vi "运维调试_CODMn.vi"() -> ()   [LabVIEW 2016, in "斯坦道CODMn新电路板.lvlib"]
uses:
  <vilib>/Utility/miscctls.llb/LVPointTypeDef.ctl
  <vilib>/Waveform/WDTFileIO.llb/Read Waveform from File.vi
  <vilib>/Utility/config.llb/NI_LVConfig.lvlib
  <vilib>/ptbypt/NI_PtbyPt.lvlib
panel:
  out "权限等级":string
  out "总步数":i32
  out "滑动杆":u8(slide) caption="测试进度" scale=0.0..100.0
  in  "参数查询":bool
  in  "仪器校准":bool
  out "仪器版本号":string
  in  "试剂余量设置":bool
  out "试剂余量显示":sgl[][](graph)
  in  "公式切换阈值滴定数(0~9999)":dbl
  out "X0":u16
  in  "平台反控标样校准":enum16{"标液1", "标液2", "标液3"}(ring)
  in  "平台反控校准量程":enum16{"低量程1", "低量程2", "高量程1", "高量程2"}(ring)
  out "注射泵保温温度":sgl format="%#.2g"
  out "量程参数显示":T1 {"(高->低)" format="%#.6g"; "阈值(低->高)" format="%#.6g"; "下限" format="%#.6g"; "上限" format="%#.6g"}
  in  "历史波形 2":bool
  in  "返回 3":bool
  out "时间-温度":u16[](array[numeric]) caption="数组"
  out "温度波形时间":timestamp
  out "ORP滴定曲线 2":u16[](graph)
  in  "历史波形":bool
  in  "返回 2":bool
  out "滴定数-ORP值":u16[](array[numeric]) caption="数组"
  out "波形时间":timestamp
  out "ORP滴定曲线":u16[](graph)
  in  "滴定曲线":bool
  out "终点滴定数":sgl format="%#.2f"
  in  "量程参数设置":bool
  out "单位:":T2(ring)
  out "运行状态":T3 {"数据时间:" format="%<%y/%m/%d %H:%M:%S>T"; "仪器时间:" format="%<%y/%m/%d %H:%M:%S>T"}
  out "模块版本号":string
  in  "模型选择":cluster{"参数":u8, "测量模式":u8, "量程":u8}
  in  "校准完毕":bool
  in  "校准按钮":T4
  in  "曲线模型":T5={"标液浓度1"=0.0, "测量吸光度1"=0.0, "样品1启用"=FALSE, "标液浓度2"=0.0, "测量吸光度2"=0.0, "样品2启用"=FALSE, "标液浓度3"=0.0, "测量吸光度3"=0.0, "样品3启用"=FALSE, "标液浓度4"=0.0, "测量吸光度4"=0.0, "样品4启用"=FALSE, "标液浓度5"=0.0, "测量吸光度5"=0.0, "样品5启用"=FALSE, "模型"=enum."线性", "method"=enum."最小二乘", "精度"=7.0, "XY图"=[], "拟合公式"="", "r^2"=0.0, "零点校准时间"=timestamp(0 s since 1904-01-01), "标液校准时间1"=timestamp(0 s since 1904-01-01), "标液校准时间2"=timestamp(0 s since 1904-01-01), "标液校准时间3"=timestamp(0 s since 1904-01-01), "标液校准时间4"=timestamp(0 s since 1904-01-01)} {"标液校准时间4" format="%<%Y/%m/%d %H:%M:%S>T"; "标液校准时间3" format="%<%Y/%m/%d %H:%M:%S>T"; "标液校准时间2" format="%<%Y/%m/%d %H:%M:%S>T"; "标液校准时间1" format="%<%Y/%m/%d %H:%M:%S>T"; "零点校准时间" format="%<%Y/%m/%d %H:%M:%S>T"; "r^2" format="%.7g"; "标液浓度5" format="%#.2f"; "测量吸光度5" format="%#.0f"; "标液浓度4" format="%#.2f"; "测量吸光度4" format="%#.0f"; "标液浓度3" format="%#.2f"; "测量吸光度3" format="%#.0f"; "标液浓度2" format="%#.2f"; "测量吸光度2" format="%#.0f"; "测量吸光度1" format="%#.0f"; "标液浓度1" format="%#.2f"}
  out "公式、校准输出":T6={"公式"={"X^2"=0.0, "X"=nan, "B"=nan}, "校准"={"校准？"=FALSE, "校准点1-5"=0, "校准浓度"=0.0}}
  out "当前步骤剩余时间":sgl format="%#.2f"
  out "加热实时温度":sgl format="%#.2f"
  out "ORP值":sgl format="%#.2f"
  in  "布尔":bool
  in  "关键参数设置":bool
  in  "流程固件":bool
  in  "模块启用":bool
  in  "串口设置":bool
  in  "公式单个写入":bool
  in  "流程路径":path=path "C:/Users/STD/Documents/斯坦道流程文件/流程.xml"
  out "字符串":string
  out "运行时间":sgl format="%#.2g"
  out "环境湿度":sgl format="%#.2g"
  out "环境温度":sgl format="%#.2g"
  out "固件版本号":string
  in  "数组":string[](array[string])
  in  "量程切换阈值写入":bool
  in  "量程切换阈值读取":bool
  in  "参数下拉列表":enum16{"CODMn"}(ring)
  in  "量程下拉列表":enum16{"低量程1", "低量程2", "高量程1", "高量程2"}(ring)
  in  "测量模式下拉列表":T7(ring)=enum."水样测量"
  in  "公式":cluster{"X^2":dbl, "X":dbl, "b":dbl}
  in  "写公式":bool
  in  "读公式":bool
  in  "返回":bool
  in  "设置":bool
  out "集成报警信息":string
  in  "定时启动":cluster{"启动":bool, "控制命令":T8, "测量参数":T9}(xcontrol)
  in  "停止":bool
  in  "手动启动":bool
  in  "单步测试":bool
  out "当前滴定数":sgl format="%#.2f"
  out "K":sgl format="%#.2f"
  out "B":sgl format="%#.2f"
  out "A":sgl format="%#.2f"
  out "多列列表框":i32(listbox)
  # "."
  # "校准时间"
  # "标液浓度"
  # "滴定数显示"
  # "标液1"
  # "标液2"
  # "标液3"
  # "零点"
  # "跨度"
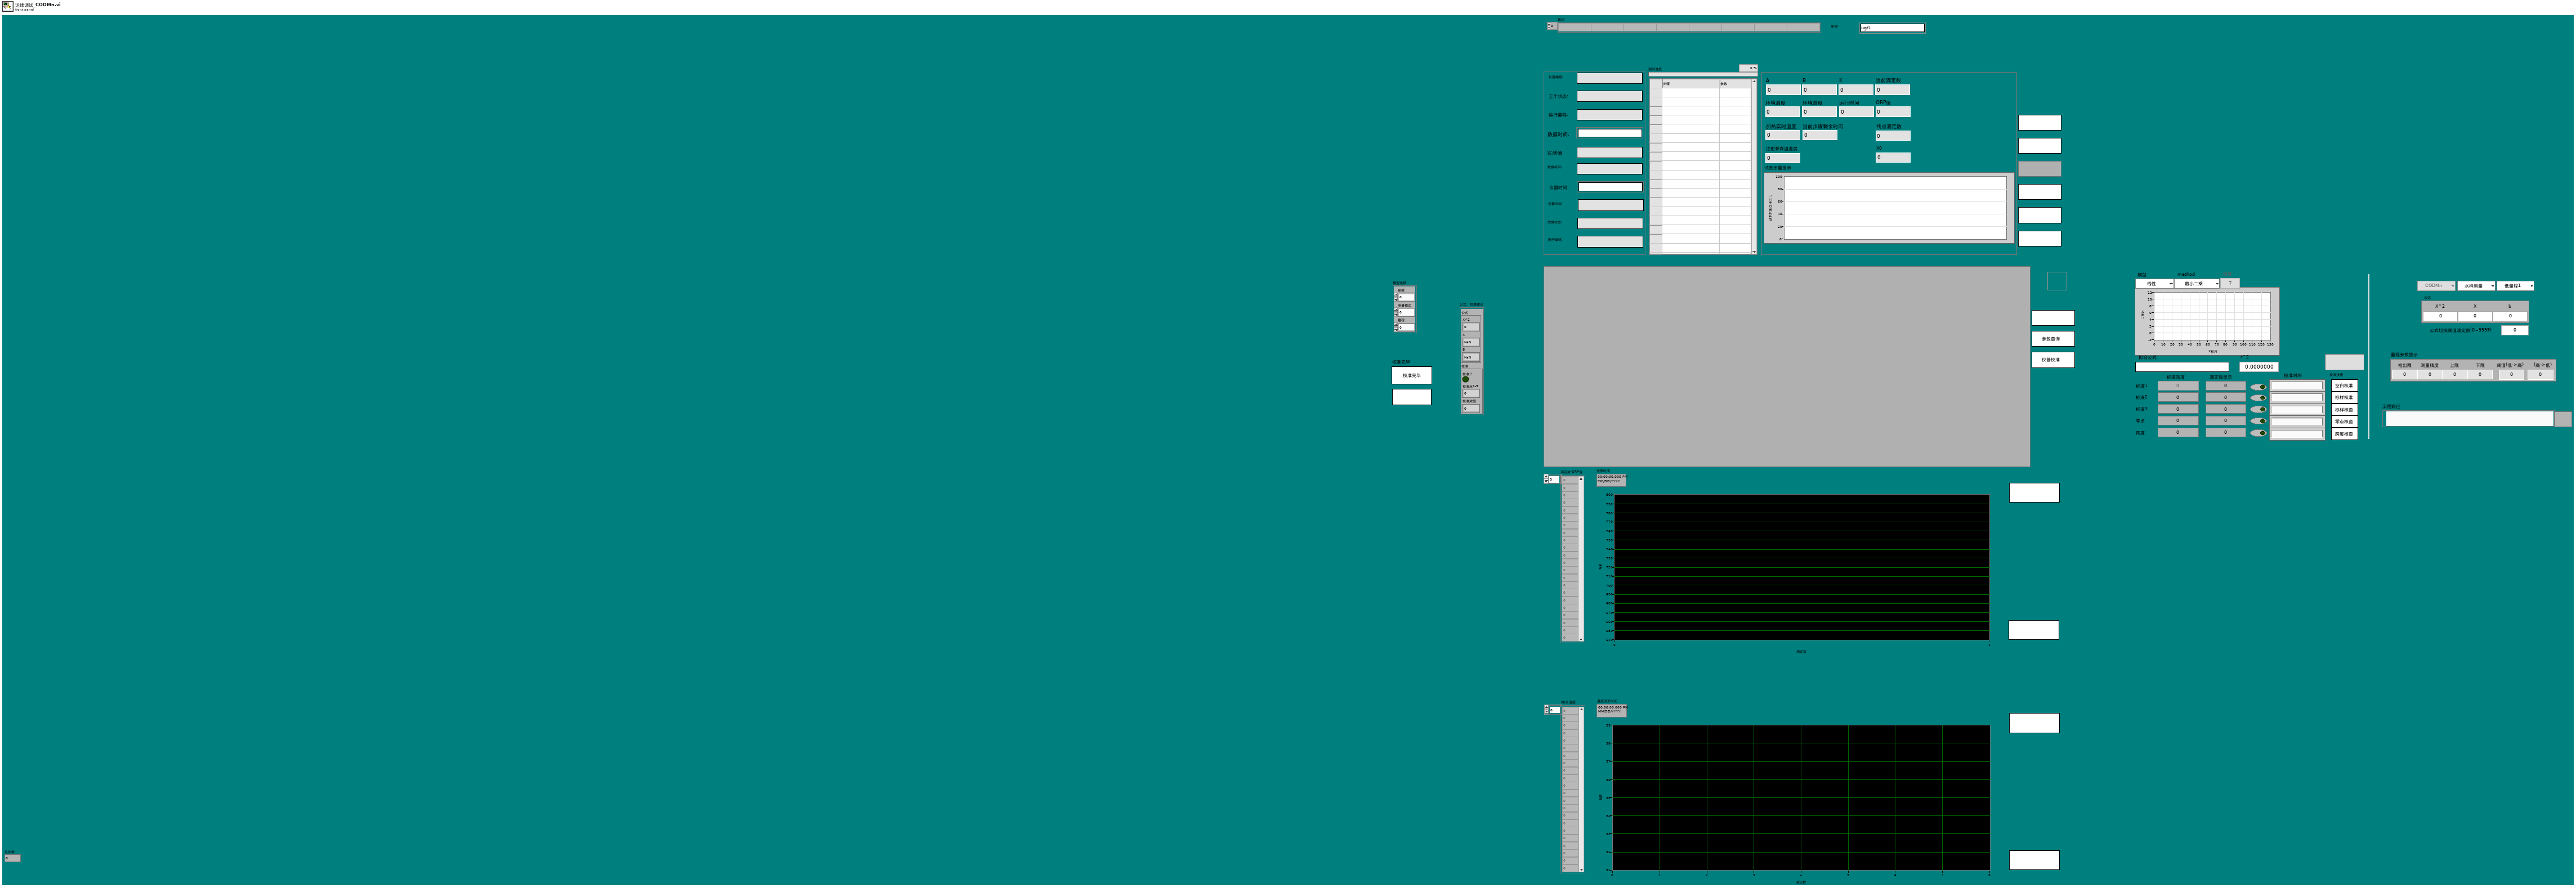
[diagram p1: front panel]
types:
  T1 = cluster{"检出限":dbl, "测量精度":dbl, "上限":dbl, "下限":dbl, "阈值(低->高)":dbl, "(高->低)":dbl}
  T2 = enum16{"ug/L", "mg/L", "ppm", "mg/m3", "cm", "ppb", "ug/m3", "%", "nmol/mol", "umol/mol", "MPN/L", "MPN/100ml", "ng/m3", "NTU", "无量纲", "ms/cm", "us/cm", "℃", "mV", "万个/L"}
  T3 = cluster{"仪器编号:":string, "工作状态:":string, "运行量程: ":string, "数据时间:":timestamp, "实测值:":string, "数据标识: ":string, "仪器时间:":timestamp, "告警状态: ":string, "故障状态:  ":string, "因子编码:":string}
  T4 = cluster{"校准1":bool, "校准2":bool, "校准3":bool, "校准4":bool, "校准5":bool}
  T5 = cluster{"标液浓度1":dbl, "测量吸光度1":dbl, "样品1启用":bool, "标液浓度2":dbl, "测量吸光度2":dbl, "样品2启用":bool, "标液浓度3":dbl, "测量吸光度3":dbl, "样品3启用":bool, "标液浓度4":dbl, "测量吸光度4":dbl, "样品4启用":bool, "标液浓度5":dbl, "测量吸光度5":dbl, "样品5启用":bool, "模型":enum32{"线性", "多项式"}, "method":enum16{"最小二乘", "最小绝对残差", "Bisquare"}, "精度":dbl, "XY图":cluster{"X Values":dbl[], "Y Values":dbl[]}[], "拟合公式":string, "r^2":dbl, "零点校准时间":timestamp, "标液校准时间1":timestamp, "标液校准时间2":timestamp, "标液校准时间3":timestamp, "标液校准时间4":timestamp}
  T6 = cluster{"公式":cluster{"X^2":dbl, "X":dbl, "B":dbl}, "校准":cluster{"校准？":bool, "校准点1-5":u16, "校准浓度":dbl}}
  T7 = enum16{"", "水样测量", "标样核查", "零点核查", "跨度核查", "空白测试", "平行样测试", "加标回收"}
  T8 = typedef "定时设置.xctl/国标控制命令.ctl" = enum16{"启动测量", "标样核查", "零点核查", "跨度核查", "空白测试", "平行样测试", "加标回收", "空白校准", "标样校准", "初始化（清洗）", "停止测试", "仪器重启", "校时", "模式设置", "测量间隔设置"}
  T9 = typedef "定时设置.xctl/测量参数.ctl" = u16
  T10 = cluster{"曲线模型":cluster{"标液浓度1":dbl, "测量吸光度1":dbl, "样品1启用":bool, "标液浓度2":dbl, "测量吸光度2":dbl, "样品2启用":bool, "标液浓度3":dbl, "测量吸光度3":dbl, "样品3启用":bool, "标液浓度4":dbl, "测量吸光度4":dbl, "样品4启用":bool, "标液浓度5":dbl, "测量吸光度5":dbl, "样品5启用":bool, "模型":enum32{"线性", "多项式"}, "method":enum16{"最小二乘", "最小绝对残差", "Bisquare"}, "精度":dbl, "XY图":cluster{"X Values":dbl[], "Y Values":dbl[]}[], "拟合公式":string, "r^2":dbl, "零点校准时间":timestamp, "标液校准时间1":timestamp, "标液校准时间2":timestamp, "标液校准时间3":timestamp, "标液校准时间4":timestamp}, "Polynomial Coefficients":dbl[]}
  T11 = cluster{"Major":u16, "Minor":u16, "Fix":u16, "Build":u16}
  T12 = typedef "NI_LVConfig.lvlib/Config Data RefNum.ctl" = refnum<k1>
  T13 = typedef "LVPointTypeDef.ctl" = cluster{"Horizontal":i16, "Vertical":i16}
  T14 = enum32{"Bad", "Idle", "Run top level", "Running"}
  T15 = cluster{"Polynomial Coefficients[0]":dbl, "Polynomial Coefficients[1]":dbl, "Polynomial Coefficients[2]":dbl}
  T16 = cluster{"检出限":dbl, "测量精度":dbl, "上限":dbl, "下限":dbl, "阈值（低->高）":dbl, "阈值（高->低）":dbl}
  T17 = cluster{"系统时间":timestamp, "工作状态":u16, "测量模式":enum16{"待机", "连续模式", "周期模式", "定点模式", "受控模式", "手动模式"}, "告警代码":u16, "故障代码":u16, "日志代码":u16, "软件版本":u16, "A":sgl, "B":sgl, "K":sgl, "当前滴定数":sgl, "T":sgl, "H":sgl, "id":u16, "flowid":u16, "量程":u16, "加热实时温度":sgl, "当前ORP值":sgl, "运行时间":sgl, "当前步骤剩余时间":sgl, "结束滴定数":sgl, "注射泵保温温度":sgl, "匹配滴定数X0":u16, "X^2":sgl, "X":sgl, "B 2":sgl}
  T18 = cluster{"因子编码":u32, "单位":u16, "标样参考值":sgl, "水样数据时间":timestamp, "水样实测值":sgl, "水样数据标识":string, "标样数据时间":timestamp, "标样实测值":sgl, "标样数据标识":string, "空白数据时间":timestamp, "空白实测值":sgl, "空白数据标识":string, "零点核查数据时间":timestamp, "零点核查实测值":sgl, "零点核查数据标识":string, "跨度核查数据时间":timestamp, "跨度核查实测值":sgl, "跨度核查数据标识":string, "加标回收数据时间":timestamp, "加标回收实测值":sgl, "加标回收数据标识":string, "平行样数据时间":timestamp, "平行样实测值":sgl, "平行样数据标识":string, "F0":sgl, "F1":sgl, "F2":sgl, "F3":sgl, "F4":sgl, "F5":sgl, "F6":sgl, "F7":sgl, "温度":sgl, "湿度":sgl, "X值":sgl, "fidrange":u16}
  T19 = cluster{"时间标识":timestamp, "设备":string, "日志信息":string, "流程参数":string}
  T20 = cluster{"时间标识":timestamp, "设备":string, "日志信息":string, "备注":string}
  T21 = typedef "LVRowAndColumnUnsignedTypeDef.ctl" = cluster{"Row":u32, "Column":u32}
  T22 = enum8{"Enabled", "Disabled", "Disabled and Grayed Out"}
  T23 = cluster{"时间源选择":enum16{"系统时间源", "仪器时间源"}, "外部时间源":timestamp}
  T24 = enum16{"空闲", "水样测试", "标样核查", "零点核查", "跨度核查", "空白测试", "平行样测试", "加标回收", "空白校准", "标样校准", "初始化（清洗）"}
  T25 = cluster{"站号":u16, "量程切换":enum32{"H", "L", "AUTO"}, "控制命令":u16, "模式设置":enum16{"待机", "连续模式", "周期模式", "定点模式", "受控模式", "手动模式"}, "测量间隔":u16}
  T26 = cluster{"参数下拉列表":enum16{"CODMn"}, "测量模式下拉列表":enum16{"", "水样测量", "标样核查", "零点核查", "跨度核查", "空白测试", "平行样测试", "加标回收"}, "量程下拉列表":enum16{"低量程1", "低量程2", "高量程1", "高量程2"}}
  T27 = cluster{"测量量程":dbl, "测量精度":dbl, "测量间隔":dbl, "消解温度":dbl, "消解时长":dbl, "空白校准时间":timestamp, "曲线截距":dbl, "曲线斜率":dbl, "测量检出限":dbl, "测量信号值":dbl, "线性相关系数":dbl, "二次多项式系数":dbl, "标样校准时间":timestamp, "稀释倍数":dbl, "三项式系数":dbl, "空白标定系数":dbl, "量程系数":dbl, "F0/ORPA":dbl, "F1/ORPB":dbl, "F2/ORPK":dbl, "F3":dbl, "F4":dbl, "F5":dbl, "F6":dbl, "F7":dbl, "X0/滴定数":dbl, "量程":dbl}
  T28 = typedef "量程选择控件.ctl" = enum32{"L", "H", "AUTO"}
  T29 = cluster{"水样测试量程模式":T28, "标样核查量程模式":T28, "零点核查量程模式":T28, "跨度核查量程模式":T28, "空白测试量程模式":T28, "平行样测试量程模式":T28, "加标回收量程模式":T28, "空白校准量程模式":T28, "标样校准量程模式":T28}
  T30 = cluster{"跨度值":dbl, "零点标准液浓度":dbl, "跨度标准液浓度":dbl, "标准液标准浓度":dbl}
  T31 = cluster{"水样测试量程模式":T28, "标样核查量程模式":T28, "零点核查量程模式":T28, "跨度核查量程模式":T28, "空白测试量程模式":T28, "平行样测试量程模式":T28, "加标回收量程模式":T28, "标样校准量程模式":T28, "空白校准量程模式":T28}
  T32 = cluster{"确定":bool, "跨度值":dbl, "零点标准液浓度":dbl, "跨度标准液浓度":dbl, "标准液标准浓度":dbl}
  T33 = cluster{"确定":bool, "测量量程":dbl, "测量精度":dbl, "测量间隔":dbl, "消解温度":dbl, "消解时长":dbl, "空白校准时间":timestamp, "曲线截距":dbl, "曲线斜率":dbl, "测量检出限":dbl, "测量信号值":dbl, "线性相关系数":dbl, "二次多项式系数":dbl, "标样校准时间":timestamp, "稀释倍数":dbl, "三项式系数":dbl, "空白标定系数":dbl, "量程系数":dbl, "F0/ORPA":dbl, "F1/ORPB":dbl, "F2/ORPK":dbl, "F3":dbl, "F4":dbl, "F5":dbl, "F6":dbl, "F7":dbl, "X0/滴定数":dbl, "量程":dbl}
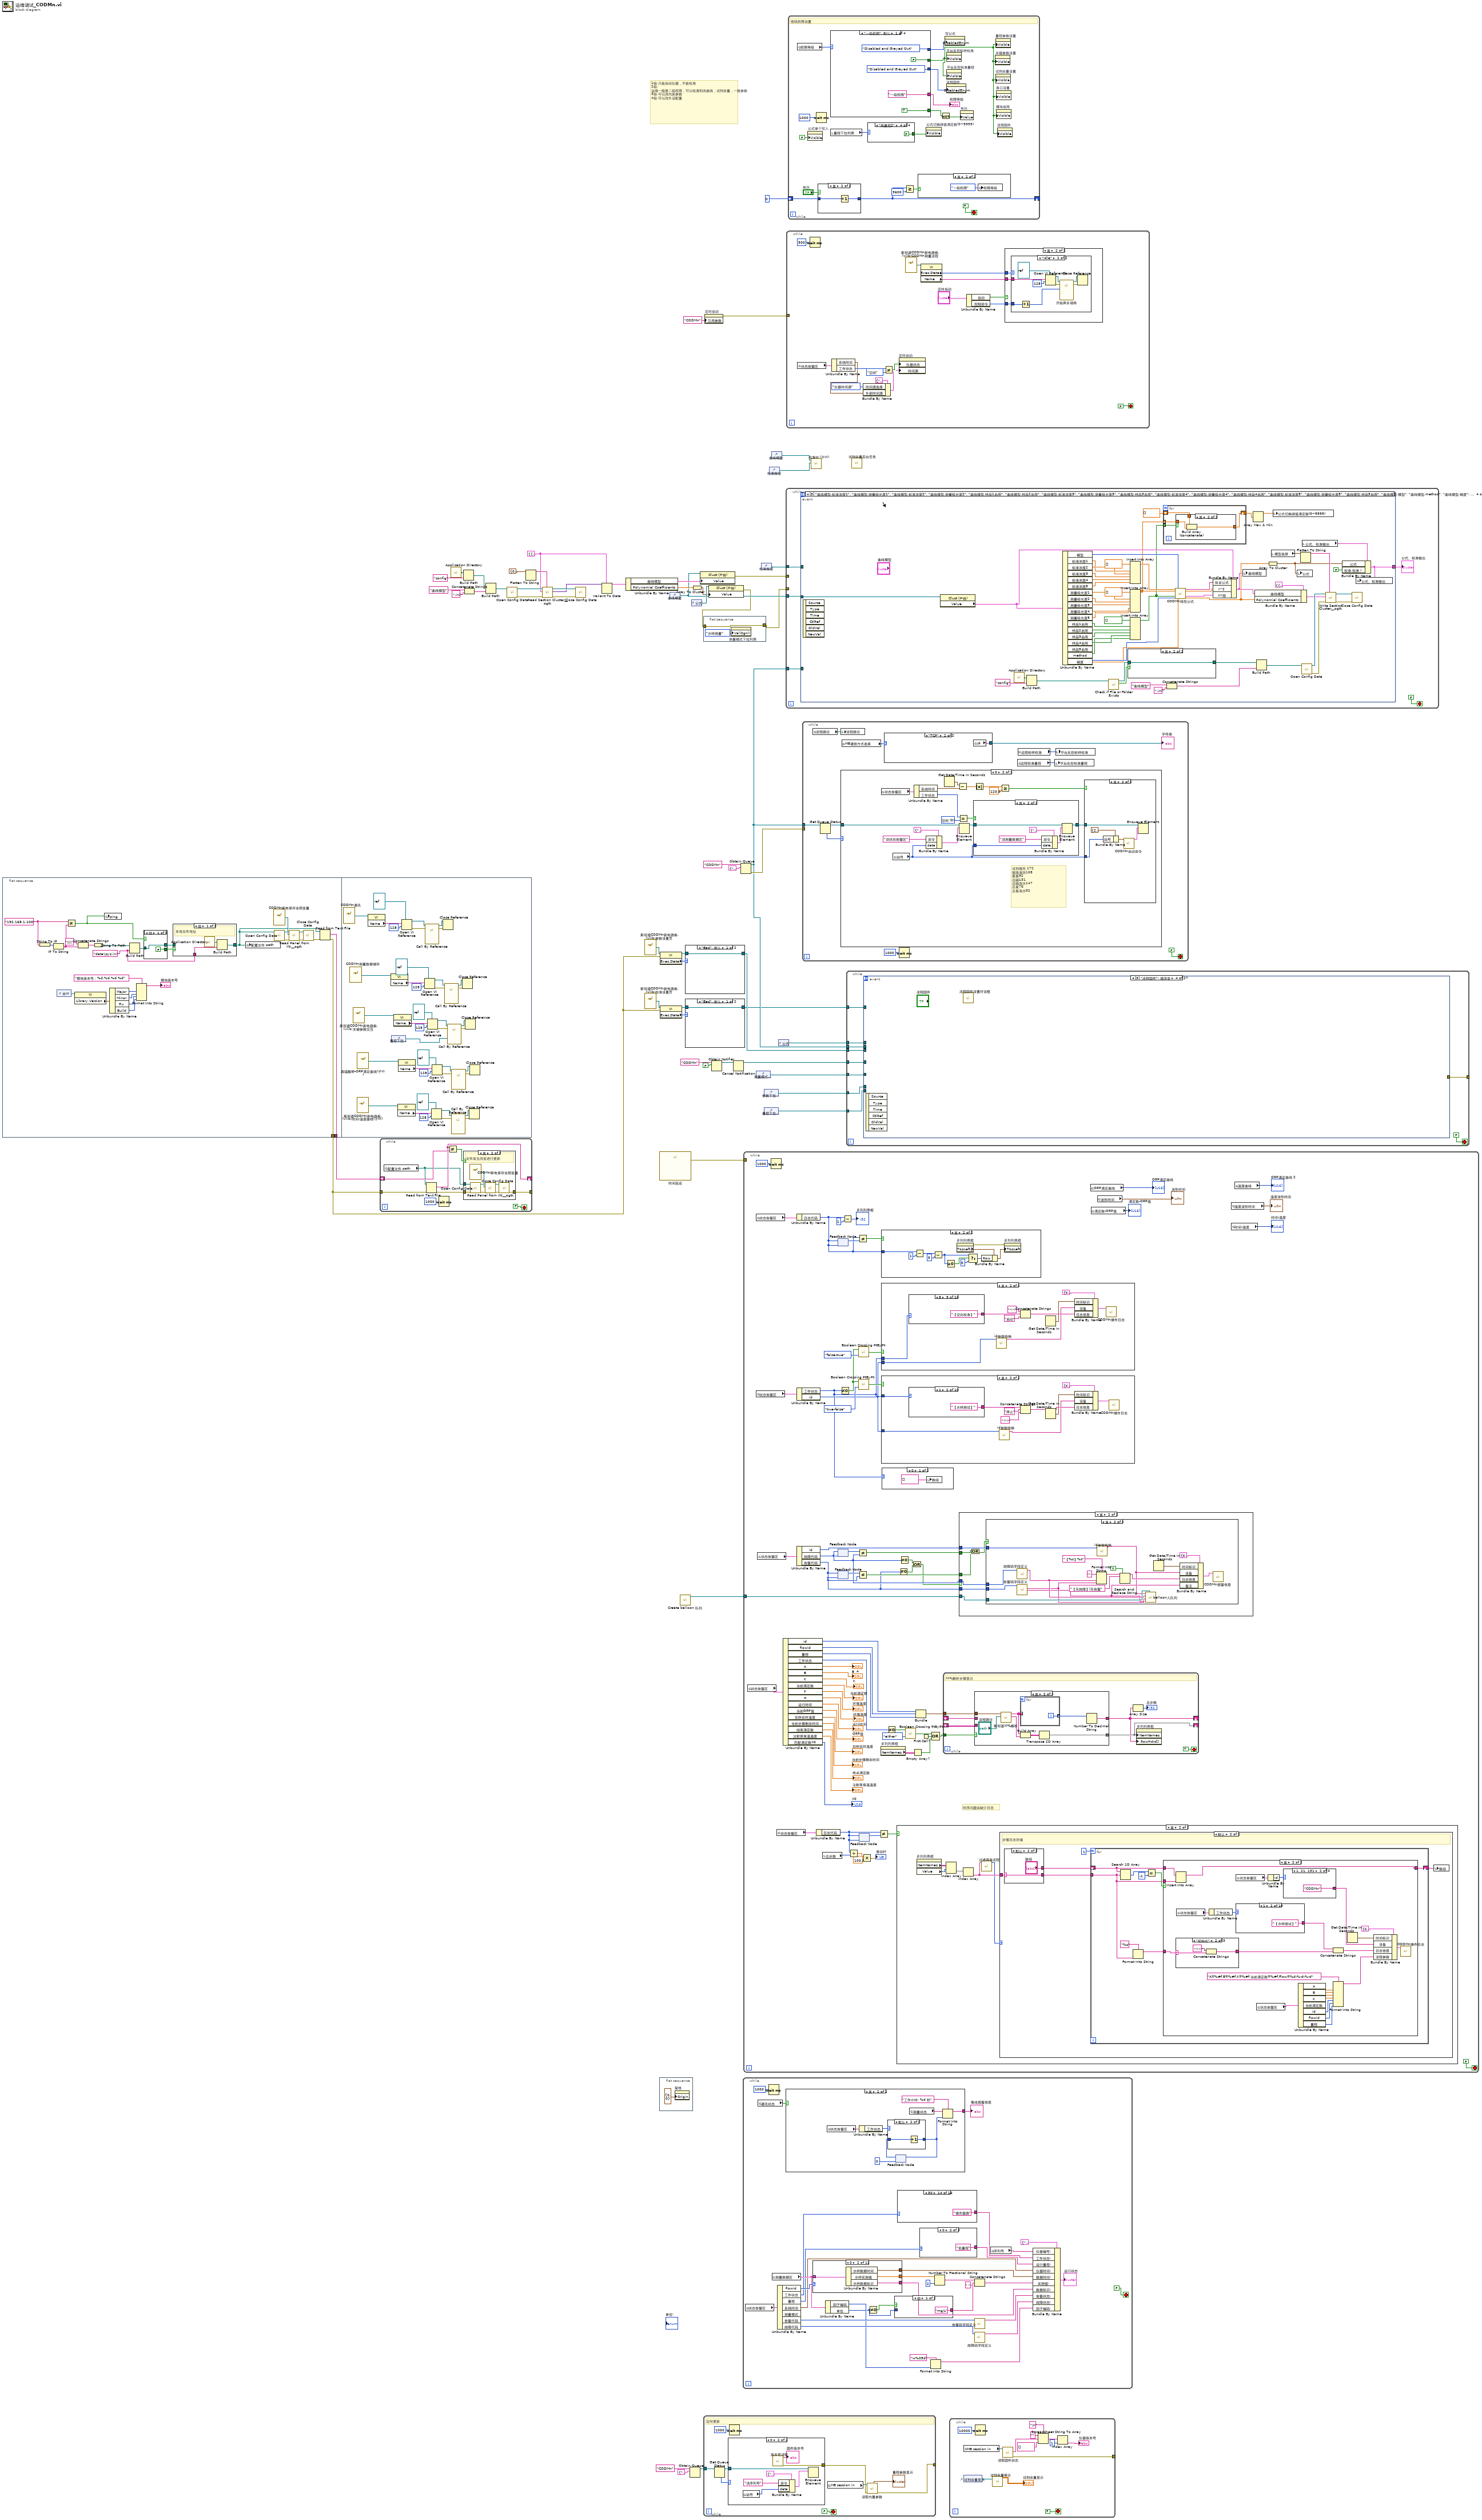
[diagram p0: block diagram]
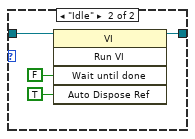
[diagram p2: hidden frame]
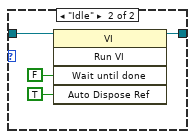
[diagram p3: hidden frame]
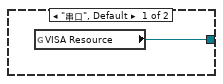
[diagram p8: hidden frame]
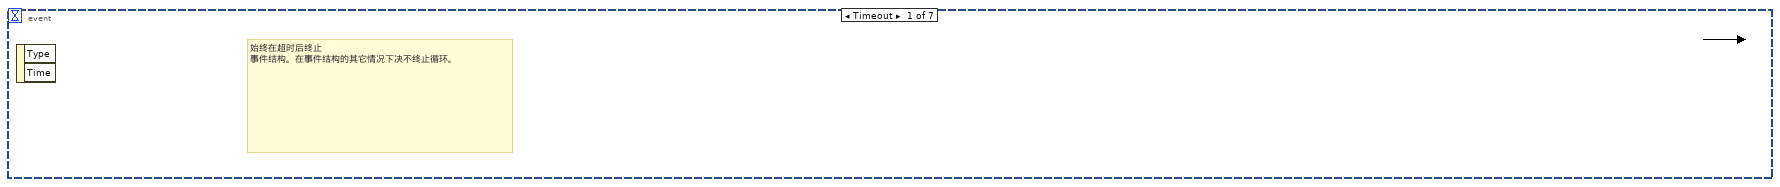
[diagram p12: hidden frame]
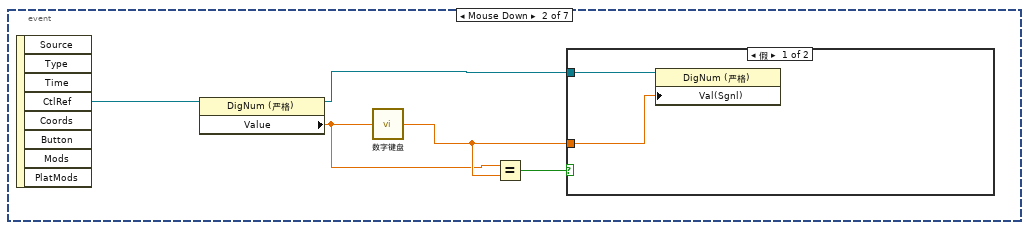
[diagram p13: hidden frame]
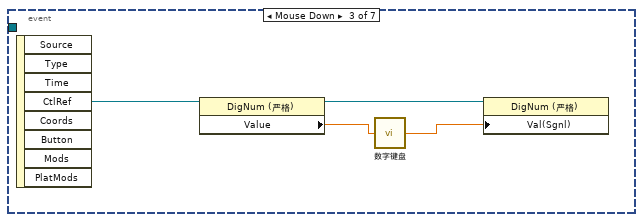
[diagram p15: hidden frame]
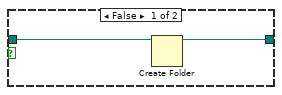
[diagram p17: hidden frame]
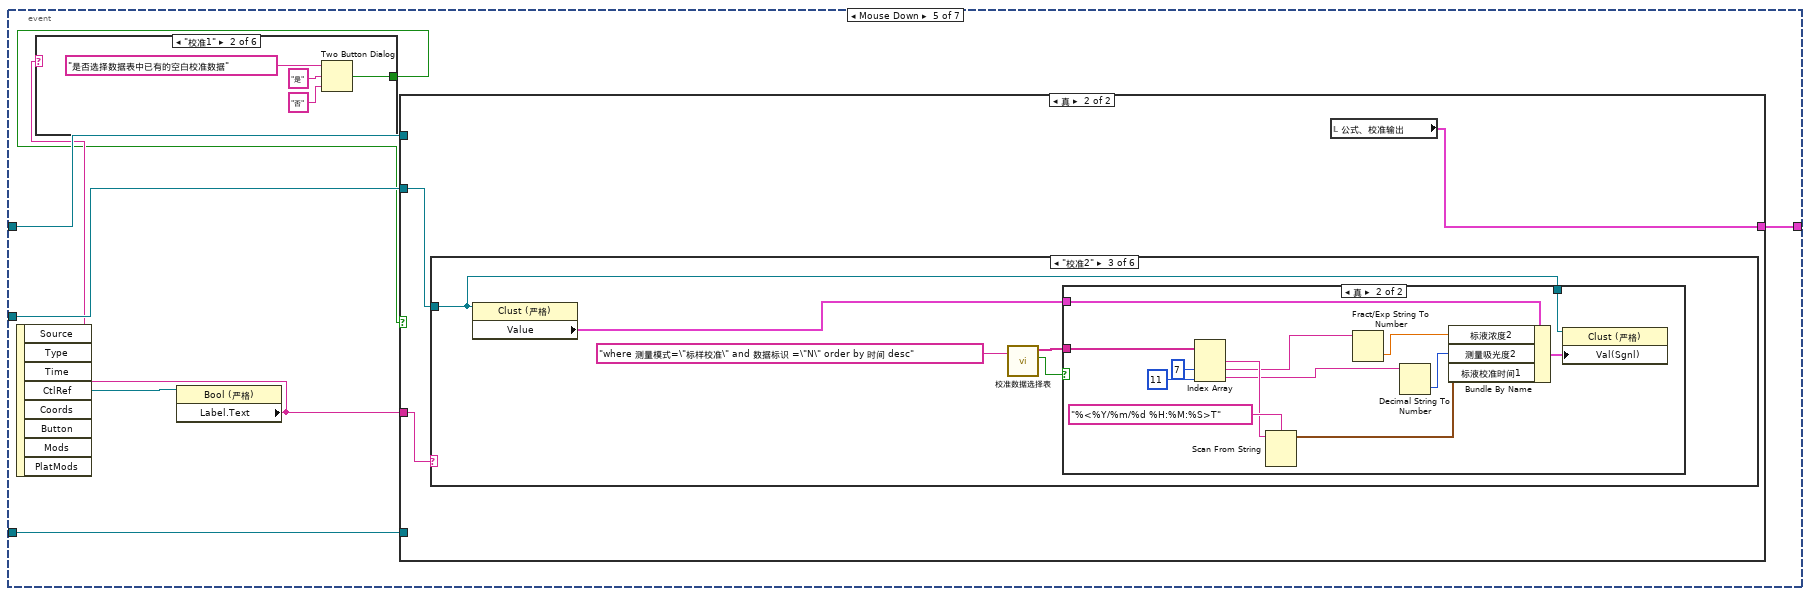
[diagram p18: hidden frame]
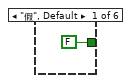
[diagram p19: hidden frame]
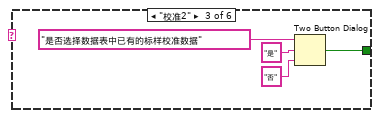
[diagram p20: hidden frame]
diagram:
  w24 = T10 {"曲线模型"={"标液浓度1"=0.0, "测量吸光度1"=0.0, "样品1启用"=FALSE, "标液浓度2"=0.0, "测量吸光度2"=0.0, "样品2启用"=FALSE, "标液浓度3"=0.0, "测量吸光度3"=0.0, "样品3启用"=FALSE, "标液浓度4"=0.0, "测量吸光度4"=0.0, "样品4启用"=FALSE, "标液浓度5"=0.0, "测量吸光度5"=0.0, "样品5启用"=FALSE, "模型"=enum."线性", "method"=enum."最小二乘", "精度"=7.0, "XY图"=[], "拟合公式"="", "r^2"=0.0, "零点校准时间"=timestamp(0 s since 1904-01-01), "标液校准时间1"=timestamp(0 s since 1904-01-01), "标液校准时间2"=timestamp(0 s since 1904-01-01), "标液校准时间3"=timestamp(0 s since 1904-01-01), "标液校准时间4"=timestamp(0 s since 1904-01-01)}, "Polynomial Coefficients"=[]} ("输出簇")
  # "1级.只能启动仪器，不能校准\n2级.运维一般是二级权限，可以校准和改曲线，试剂余量，一般参数\n3级.可以改内部参数\n4级.可以改外设配置"
  n1 = flat-sequence {
    tunnel: [w59] -> w1
    tunnel: [w58] -> w41
    frame #0 {
      w79 = "data\\sys.ini" ("名称或相对路径")
      w71 = "192.168.1.100" ("名称")
      n2 = String To IP(1:w71) -> (0:w78:u32)
      n3 = IP To String(2:w78) -> (0:w75:string)  [unwired: 1 in]
      n4 = control-ref of="本VI"() -> (w69:refnum<vi>)
      n5 = Not Equal?(x=w71, y=w75) -> (x != y?=w80:bool)
      n6 = property class="VI"(reference=w69) -> ("Library.Version"=w68:T11)  [unwired: 1 in, 2 out]
      n7 = Concatenate Strings("\\\\" ("字符串"), w75) -> (w76:string)
      n8 = String To Path(string=w76) -> (path=w70:path)
      n9 = global write "VARCODMn全局变量.vi" "ping"(w80) -> ()
      n10 = Unbundle By Name(w68) -> ("Major"=w66:u16, "Minor"=w65:u16, "Fix"=w64:u16, "Build"=w63:u16)
      n11 = Build Path(base path=w70, name or relative path=w79) -> (appended path=w74:path)
      n12 = Format Into String(format string="模块版本号：%d.%d.%d.%d" ("格式字符串"), w66, w65, w64, w63) -> (resulting string=→"模块版本号":string)  [unwired: 2 in, 1 out]
      n13 = case shown="假" w80 {
        tunnel: w74 -> [w86 w90]
        tunnel: [w86 w89] -> w73
        tunnel: [FALSE w88] -> w72
        frame False {
        }
        frame True {
          n14 = call <vilib>:"Check if File or Folder Exists.vi"("path"=w90) -> ("file or folder exists?"=w88:bool, "dup path"=w89:path)  [unwired: 8 in, 1 out]
        }
      }
      n15 = case shown="假" w72 {
        tunnel: w73 -> [_ w94]
        tunnel: [w92 w94] -> w61
        tunnel: w79 -> [w91 _]
        frame False {
          # "本地文件地址"
          n16 = call <vilib>:"Application Directory.vi"() -> ("Application Directory"=w93:path)
          n17 = Build Path(base path=w93, name or relative path=w91) -> (appended path=w92:path)
        }
        frame True {
          # "网络共享地址"
        }
      }
      n18 = global write "VARCODMn全局变量.vi" "配置文件 path"(w61) -> ()
      n19 = vi-ref "CODMn断电保存全局变量.vi"() -> (w84:refnum<vi>)
      n20 = call <vilib>:"Open Config Data.vi"("configuration file path"=w61) -> ("error out"=w82:errorcluster, "refnum"=w85:T12)  [unwired: 8 in, 1 out]
      n21 = call <userlib>:"Read Panel from INI__ogtk.vi"("error in (no error)"=w82, "VI ref"=w84, "refnum"=w85) -> ("error out"=w81:errorcluster, "refnum out"=w83:T12)  [unwired: 7 in]
      n22 = call <vilib>:"Close Config Data.vi"("error in (no error)"=w81, "refnum"=w83) -> ("error out"=w60:errorcluster)  [unwired: 8 in, 1 out]
      n23 = Read from Text File(file (use dialog)=w61, error in=w60) -> (text=w58:string, error out=w59:errorcluster)  [unwired: 2 in, 2 out]
    }
    frame #1 {
      n24 = vi-ref "CODMn通讯.vi"() -> (w103:refnum<vi>)
      n25 = vi-ref "CODMn测量数据储存.vi"() -> (w135:refnum<vi>)
      n26 = vi-ref "斯坦道CODMn新电路板.lvlib:关键参数交互.vi"() -> (w121:refnum<vi>)
      n27 = vi-ref "斯坦道CODMn新电路板.lvlib:时间-温度曲线(子VI).vi"() -> (w105:refnum<vi>)
      n28 = vi-ref "高锰酸钾-ORP滴定曲线(子VI).vi"() -> (w118:refnum<vi>)
      n29 = property class="VI"(reference=w103) -> ("Name"=w102:string)  [unwired: 1 in, 2 out]
      n30 = property class="VI"(reference=w135) -> ("Name"=w128:string)  [unwired: 1 in, 2 out]
      n31 = control-ref of="量程下拉列表"() -> (w95:refnum<vi>)
      n32 = property class="VI"(reference=w121) -> ("Name"=w127:string)  [unwired: 1 in, 2 out]
      n33 = property class="VI"(reference=w105) -> ("Name"=w111:string)  [unwired: 1 in, 2 out]
      n34 = property class="VI"(reference=w118) -> ("Name"=w112:string)  [unwired: 1 in, 2 out]
      n35 = Open VI Reference(type specifier VI Refnum (for type only)=refnum<vi> refnum, vi path=w102, options=128 ("选项")) -> (vi reference=w100:refnum<vi>, error out=w98:errorcluster)  [unwired: 3 in]
      n36 = Open VI Reference(type specifier VI Refnum (for type only)=refnum<vi> refnum, vi path=w128, options=128 ("选项")) -> (vi reference=w130:refnum<vi>, error out=w132:errorcluster)  [unwired: 3 in]
      n37 = call-by-ref "?"(reference=w100, error in=w98) -> (reference out=w96:refnum<vi>, error out=w97:errorcluster)  [unwired: 12 in]
      n38 = Open VI Reference(type specifier VI Refnum (for type only)=refnum<vi> refnum, vi path=w127, options=128 ("选项")) -> (vi reference=w125:refnum<vi>, error out=w124:errorcluster)  [unwired: 3 in]
      n39 = Open VI Reference(type specifier VI Refnum (for type only)=refnum<vi> refnum, vi path=w111, options=128 ("选项")) -> (vi reference=w109:refnum<vi>, error out=w108:errorcluster)  [unwired: 3 in]
      n40 = Open VI Reference(type specifier VI Refnum (for type only)=refnum<vi> refnum, vi path=w112, options=128 ("选项")) -> (vi reference=w114:refnum<vi>, error out=w115:errorcluster)  [unwired: 3 in]
      n41 = Close Reference(reference=w96, error in (no error)=w97) -> ()  [unwired: 1 out]
      n42 = call-by-ref "?"(reference=w130, error in=w132) -> (reference out=w134:refnum<vi>, error out=w133:errorcluster)  [unwired: 12 in]
      n43 = call-by-ref "?"(reference=w125, error in=w124, "量程下拉列表"=w95) -> (reference out=w122:refnum<vi>, error out=w123:errorcluster)  [unwired: 11 in]
      n44 = call-by-ref "?"(reference=w109, error in=w108) -> (reference out=w106:refnum<vi>, error out=w107:errorcluster)  [unwired: 12 in]
      n45 = call-by-ref "?"(reference=w114, error in=w115) -> (reference out=w117:refnum<vi>, error out=w116:errorcluster)  [unwired: 12 in]
      n46 = Close Reference(reference=w134, error in (no error)=w133) -> ()  [unwired: 1 out]
      n47 = Close Reference(reference=w122, error in (no error)=w123) -> ()  [unwired: 1 out]
      n48 = Close Reference(reference=w106, error in (no error)=w107) -> ()  [unwired: 1 out]
      n49 = Close Reference(reference=w117, error in (no error)=w116) -> ()  [unwired: 1 out]
    }
  }
  n50 = while {
    tunnel: [w143] -> _
    shift-right: [w138] -> _
    shift-left: w41 -> [w141]
    tunnel: w1 -> [w139]
    stop <- FALSE stop-if-true
    n51 = global read "VARCODMn全局变量.vi" "配置文件 path"() -> (w136:path)
    n52 = Read from Text File(file (use dialog)=w136, error in=w139) -> (text=w138:string, error out=w137:errorcluster)  [unwired: 2 in, 2 out]
    n53 = Wait (ms)(milliseconds to wait=u32 1000 ("等待时间（毫秒）")) -> ()  [unwired: 1 out]
    n54 = Not Equal?(x=w138, y=w141) -> (x != y?=w140:bool)
    n55 = case shown="真" w140 {
      tunnel: [w145 w149] -> w143
      tunnel: w136 -> [_ w148]
      tunnel: w137 -> [w145 w147]
      frame False {
      }
      frame True {
        # "文件发生改变进行更新"
        n56 = vi-ref "CODMn断电保存全局变量.vi"() -> (w146:refnum<vi>)
        n57 = call <vilib>:"Open Config Data.vi"("error in (no error)"=w147, "configuration file path"=w148) -> ("error out"=w153:errorcluster, "refnum"=w152:T12)  [unwired: 7 in, 1 out]
        n58 = call <userlib>:"Read Panel from INI__ogtk.vi"("error in (no error)"=w153, "VI ref"=w146, "refnum"=w152) -> ("error out"=w151:errorcluster, "refnum out"=w150:T12)  [unwired: 7 in]
        n59 = call <vilib>:"Close Config Data.vi"("error in (no error)"=w151, "refnum"=w150) -> ("error out"=w149:errorcluster)  [unwired: 8 in, 1 out]
      }
    }
  }
  n60 = call <vilib>:"Application Directory.vi"() -> ("Application Directory"=w34:path)
  n61 = Build Path(base path=w34, name or relative path="config" ("名称或相对路径")) -> (appended path=w32:path)
  n62 = Concatenate Strings("曲线模型" ("字符串"), ".ini" ("字符串")) -> (w30:string)
  n63 = Build Path(base path=w32, name or relative path=w30) -> (appended path=w35:path)
  n64 = call <vilib>:"Open Config Data.vi"("configuration file path"=w35) -> ("error out"=w38:errorcluster, "refnum"=w39:T12)  [unwired: 8 in, 1 out]
  n65 = Flatten To String(anything=cluster{"参数":u8, "测量模式":u8, "量程":u8} {"参数"=0, "测量模式"=0, "量程"=0} ("模型选择")) -> (data string=w28:string)  [unwired: 3 in, 2 out]
  n66 = call <userlib>:"Read Section Cluster__ogtk.vi"("section (optional)"=w28, "error in (no error)"=w38, "Section Formatted Cluster Type"=w24, "refnum"=w39) -> ("error out"=w36:errorcluster, "Section Formatted Cluster"=w29:variant, "dup refnum"=w37:T12)  [unwired: 3 in, 2 out]
  n67 = call <vilib>:"Close Config Data.vi"("error in (no error)"=w36, "refnum"=w37) -> ()  [unwired: 8 in, 2 out]
  n68 = Variant To Data(type=w24, Variant=w29) -> (data=w26:T10)  [unwired: 1 in, 1 out]
  n69 = Unbundle By Name(w26) -> ("曲线模型"=w25:T5, "Polynomial Coefficients"=w23:dbl[])
  n70 = vi-ref "斯坦道CODMn新电路板.lvlib:参数设置页.vi"() -> (w6:refnum<vi>)
  n71 = vi-ref "斯坦道CODMn新电路板.lvlib:校准设置页.vi"() -> (w9:refnum<vi>)
  n72 = call "时间延迟"() -> ("error out"=w50:errorcluster)  [unwired: 11 in]
  n73 = flat-sequence {
    frame #0 {
      n74 = property on="窗格" class="Pane"("Origin"=T13 {"Horizontal"=0, "Vertical"=0} ("原点")) -> ()  [unwired: 2 in, 2 out]
    }
  }
  n75 = property class="VI"(reference=w6, error in=w1) -> (reference out=w4:refnum<vi>, "Exec.State"=w5:T14)  [unwired: 1 out]
  n76 = property class="VI"(reference=w9, error in=w1) -> (reference out=w7:refnum<vi>, "Exec.State"=w8:T14)  [unwired: 1 out]
  n77 = control-ref of="曲线模型"() -> (w21:refnum<vi>)
  n78 = call "Create balloon 队列.vi"() -> ("队列输出"=w40:refnum<queue>)  [unwired: 11 in]
  n79 = case shown="\"Bad\", 默认" w5 {
    tunnel: w4 -> [w155 w159]
    tunnel: [w155 w156] -> w3
    frame "Bad", Default {
    }
    frame "Idle" {
      n80 = invoke class="VI" method="Run VI"(reference=w159, "Wait until done"=FALSE ("结束前等待"), "Auto Dispose Ref"=TRUE ("自动销毁引用")) -> (reference out=w156:refnum<vi>)  [unwired: 2 in, 4 out]
    }
  }
  n81 = case shown="\"Bad\", 默认" w8 {
    tunnel: w7 -> [w160 w164]
    tunnel: [w160 w161] -> w2
    frame "Bad", Default {
    }
    frame "Idle" {
      n82 = invoke class="VI" method="Run VI"(reference=w164, "Wait until done"=FALSE ("结束前等待"), "Auto Dispose Ref"=TRUE ("自动销毁引用")) -> (reference out=w161:refnum<vi>)  [unwired: 2 in, 4 out]
    }
  }
  n83 = Obtain Queue(name (unnamed)="CODMn" ("名称（未命名）"), element data type=cluster{"命令":string, "data":variant} {"命令"="", "data"=variant}) -> (queue out=w14:refnum<queue>)  [unwired: 3 in, 2 out]
  n84 = control-ref of="公式"() -> (w20:refnum<vi>)
  n85 = Array To Cluster(array=w23) -> (cluster=w19:T15)
  n86 = property class="Clust (严格)"(reference=w21, "Value"=w25) -> (error out=w18:errorcluster)  [unwired: 1 in, 1 out]
  n87 = flat-sequence {
    tunnel: w11 -> [w165]
    tunnel: [w165] -> w10
    frame #0 {
      n88 = property on="测量模式下拉列表" class="Enum (严格)"("Val(Sgnl)"=T7."水样测量" ("值(信号)")) -> ()  [unwired: 2 in, 2 out]
    }
  }
  n89 = while {
    tunnel: w14 -> [w174]
    tunnel: [w167] -> _
    stop <- FALSE stop-if-true
    # "定时更新"
    n90 = Get Queue Status(queue=w174) -> (queue out=w172:refnum<queue>, # elements in queue=w171:i32)  [unwired: 2 in, 6 out]
    n91 = case shown="0" w171 {
      tunnel: [_ w179] -> w168
      tunnel: w172 -> [_ w178]
      frame Default {
      }
      frame 0 {
        n92 = global read "CODMn断电保存全局变量.vi" "站号"() -> (w177:u16)
        n93 = call "版本号读取.vi"() -> ("error out"=w179:errorcluster, "固件版本号"=→"固件版本号":string)  [unwired: 10 in]
        n94 = Bundle By Name(cluster=cluster{"命令":string, "data":variant} {"命令"="", "data"=variant} ("元素"), "命令"="读序列号", "data"=w177) -> (w180:cluster{"命令":string, "data":variant})
        n95 = Enqueue Element(queue=w178, element=w180) -> ()  [unwired: 2 in, 3 out]
      }
    }
    n96 = Wait (ms)(milliseconds to wait=u32 1000 ("等待时间（毫秒）")) -> ()  [unwired: 1 out]
    n97 = global read "VARCODMn全局变量.vi" "MB session in"() -> (w170:refnum<class "MB_Master.lvclass">)
    n98 = call "读取内置参数.vi"("error in (no error)"=w168, "MB session in"=w170) -> ("error out"=w167:errorcluster, "量程参数读取"=→"量程参数显示":T16)  [unwired: 5 in, 3 out]
  }
  n99 = property on="定时启动" class="定时设置 (严格)"("引用参数"="CODMn") -> (error out=w13:errorcluster)  [unwired: 2 in, 1 out]
  n100 = property class="Clust (严格)"(reference=w20, "Value"=w19) -> (error out=w11:errorcluster)  [unwired: 1 in, 1 out]
  n101 = Obtain Notifier(name (unnamed)="CODMn" ("名称（未命名）"), notification data type=FALSE) -> (notifier out=w47:refnum<notifier>)  [unwired: 2 in, 2 out]
  n102 = Cancel Notification(0:w47) -> (8:w46:refnum<notifier>)  [unwired: 1 in, 2 out]
  n103 = Obtain Queue(name (unnamed)="CODMn" ("名称（未命名）"), element data type=cluster{"命令":string, "data":variant} {"命令"="", "data"=variant}) -> (queue out=w44:refnum<queue>, error out=w55:errorcluster)  [unwired: 3 in, 1 out]
  n104 = while {
    stop <- FALSE stop-if-true
    n105 = global read "VARCODMn全局变量.vi" "状态告警区"() -> (w210:T17)
    n106 = global read "VARCODMn全局变量.vi" "通讯状态"() -> (w212:bool)
    n107 = Wait (ms)(milliseconds to wait=u32 1000 ("等待时间（毫秒）")) -> ()  [unwired: 1 out]
    n108 = global read "VARCODMn全局变量.vi" "测量数据区"() -> (w208:T18)
    n109 = Unbundle By Name(w210) -> ("flowid"=w209:u16, "工作状态"=w206:u16, "量程"=w204:u16, "系统时间"=w202:timestamp, "告警代码"=w192:u16, "故障代码"=w190:u16)  [unwired: 1 out]
    n110 = case shown="真" w212 {
      tunnel: ["通讯异常" ("集成报警信息") w290] -> w211
      frame False {
      }
      frame True {
        n111 = global read "VARCODMn全局变量.vi" "状态告警区"() -> (w296:T17)
        n112 = Unbundle By Name(w296) -> ("工作状态"=w295:u16)
        n113 = feedback #1(0) -> (w293:i32)
        n114 = case shown="默认" w295 {
          tunnel: w293 -> [_ w298]
          tunnel: [_ w297] -> w291
          frame 0 {
          }
          frame Default {
            n115 = Increment(x=w298) -> (x+1=w297:i32)
          }
        }
        n116 = feedback-in #1(w291) -> ()
        n117 = global read "VARCODMn全局变量.vi" "测量状态"() -> (w289:string)
        n118 = Format Into String(format string="工作计时: %d 秒" ("格式字符串"), initial string=w289, w291) -> (resulting string=w290:string)  [unwired: 1 in, 1 out]
      }
    }
    "集成报警信息" <- w211
    n119 = case shown="0" w209 {
      selector: w209 -> [w241 _ _ _ _ _ _ _ _ _ _ _]
      tunnel: [_ w247 w251 w255 w259 w263 w267 w271 w275 w278 w282 w287] -> w199
      tunnel: [_ w245 w250 w254 w258 w262 w266 w269 w274 w277 w281 w286] -> w194
      tunnel: [_ w244 w249 w253 w257 w261 w265 w268 w273 w276 w280 w285] -> w193
      tunnel: w208 -> [_ w246 w248 w252 w256 w260 w264 w270 w272 w279 w283 w284]
      frame Default {
        n120 = Format Into String(format string="%d" ("格式字符串"), initial string="未知" ("工作状态"), w241) -> ()  [unwired: 1 in, 2 out]
      }
      frame 0 {
        n121 = Unbundle By Name(w246) -> ("水样数据时间"=w247:timestamp, "水样实测值"=w245:sgl, "水样数据标识"=w244:string)
      }
      frame 1 {
        n122 = Unbundle By Name(w248) -> ("水样数据时间"=w251:timestamp, "水样实测值"=w250:sgl, "水样数据标识"=w249:string)
      }
      frame 2 {
        n123 = Unbundle By Name(w252) -> ("标样数据时间"=w255:timestamp, "标样实测值"=w254:sgl, "标样数据标识"=w253:string)
      }
      frame 3 {
        n124 = Unbundle By Name(w256) -> ("零点核查数据时间"=w259:timestamp, "零点核查实测值"=w258:sgl, "零点核查数据标识"=w257:string)
      }
      frame 4 {
        n125 = Unbundle By Name(w260) -> ("跨度核查数据时间"=w263:timestamp, "跨度核查实测值"=w262:sgl, "跨度核查数据标识"=w261:string)
      }
      frame 5 {
        n126 = Unbundle By Name(w264) -> ("空白数据时间"=w267:timestamp, "空白实测值"=w266:sgl, "空白数据标识"=w265:string)
      }
      frame 6 {
        n127 = Unbundle By Name(w270) -> ("平行样数据时间"=w271:timestamp, "平行样实测值"=w269:sgl, "平行样数据标识"=w268:string)
      }
      frame 7 {
        n128 = Unbundle By Name(w272) -> ("加标回收数据时间"=w275:timestamp, "加标回收实测值"=w274:sgl, "加标回收数据标识"=w273:string)
      }
      frame 8 {
        n129 = Unbundle By Name(w279) -> ("空白数据时间"=w278:timestamp, "空白实测值"=w277:sgl, "空白数据标识"=w276:string)
      }
      frame 9 {
        n130 = Unbundle By Name(w283) -> ("标样数据时间"=w282:timestamp, "标样实测值"=w281:sgl, "标样数据标识"=w280:string)
      }
      frame 10 {
        n131 = Unbundle By Name(w284) -> ("水样数据时间"=w287:timestamp, "水样实测值"=w286:sgl, "水样数据标识"=w285:string)
      }
    }
    n132 = Unbundle By Name(w208) -> ("因子编码"=w186:u32, "单位"=w183:u16)
    n133 = Not Equal To 0?(x=w183) -> (x != 0?=w184:bool)
    n134 = case shown="假" w184 {
      tunnel: ["mg/L" ("RingText.Text") w217] -> w188
      tunnel: w183 -> [_ w216]
      frame False {
      }
      frame True {
        n135 = property on="单位:" class="Enum (严格)"("Value"=w216) -> (error out=w218:errorcluster)  [unwired: 2 in, 1 out]
        n136 = property on="单位:" class="Enum (严格)"(error in=w218) -> ("RingText.Text"=w217:string)  [unwired: 1 in, 2 out]
      }
    }
    n137 = case shown="30" w206 {
      selector: w206 -> [w222 _ _ _ _ _ _ _ _ _ _ _ _ _ _ _]
      tunnel: [w223 "空闲" ("工作状态") "水样测量" ("工作状态") "标样核查" ("工作状态") "零点核查" ("工作状态") "跨度核查" ("工作状态") "空白测试" ("工作状态") "平行样测试" ("工作状态") "加标回收" ("工作状态") "空白校准" ("工作状态") "标样校准" ("工作状态") "初始化" ("工作状态") "调试" ("工作状态") "填充管路" ("工作状态") "清洗管路" ("工作状态") "清洗反应杯" ("工作状态")] -> w205
      frame Default {
        n138 = Format Into String(format string="%d" ("格式字符串"), initial string="未知" ("工作状态"), w222) -> (resulting string=w223:string)  [unwired: 1 in, 1 out]
      }
      frame 0 {
      }
      frame 1 {
      }
      frame 2 {
      }
      frame 3 {
      }
      frame 4 {
      }
      frame 5 {
      }
      frame 6 {
      }
      frame 7 {
      }
      frame 8 {
      }
      frame 9 {
      }
      frame 10 {
      }
      frame 22 {
      }
      frame 30 {
      }
      frame 31 {
      }
      frame 32 {
      }
    }
    n139 = case shown="0" w204 {
      tunnel: ["" ("字符串") "低量程" ("字符串") "高量程" ("字符串")] -> w203
      frame Default {
      }
      frame 0 {
      }
      frame 1 {
      }
    }
    n140 = Format Into String(format string="w%05d" ("格式字符串"), w186) -> (resulting string=w185:string)  [unwired: 2 in, 1 out]
    n141 = Number To Fractional String(number=w194, precision (6)=i16 2 ("精度(6)")) -> (F-format string=w197:string)  [unwired: 2 in]
    n142 = Concatenate Strings(w197, " " ("字符串"), w188) -> (w195:string)
    n143 = call "告警码字段定义.vi"("告警代码"=w192) -> ("字符串"=w191:string)  [unwired: 8 in, 2 out]
    n144 = call "故障码字段定义.vi"("故障代码"=w190) -> ("字符串"=w189:string)  [unwired: 10 in]
    n145 = global read "VARCODMn全局变量.vi" "序列号"() -> (w207:string)
    n146 = Bundle By Name(cluster=T3 {"仪器编号:"="", "工作状态:"="", "运行量程: "="", "数据时间:"=timestamp(0 s since 1904-01-01), "实测值:"="", "数据标识: "="", "仪器时间:"=timestamp(0 s since 1904-01-01), "告警状态: "="", "故障状态:  "="", "因子编码:"=""} ("运行状态"), "仪器编号:"=w207, "工作状态:"=w205, "运行量程:"=w203, "仪器时间:"=w202, "数据时间:"=w199, "实测值:"=w195, "数据标识:"=w193, "告警状态:"=w191, "故障状态:"=w189, "因子编码:"=w185) -> (→"运行状态":T3)
  }
  n147 = while {
    tunnel: w50 -> [_]
    tunnel: w40 -> [w321]
    stop <- FALSE stop-if-true
    # "时序问题会缺少日志"
    n148 = global read "VARCODMn全局变量.vi" "状态告警区"() -> (w359:T17)
    n149 = global read "VARCODMn全局变量.vi" "状态告警区"() -> (w324:T17)
    n150 = global read "VARCODMn全局变量.vi" "状态告警区"() -> (w346:T17)
    n151 = global read "VARCODMn全局变量.vi" "状态告警区"() -> (w350:T17)
    n152 = Wait (ms)(milliseconds to wait=u32 1000 ("等待时间（毫秒）")) -> ()  [unwired: 1 out]
    n153 = global read "VARCODMn全局变量.vi" "状态告警区"() -> (w344:T17)
    n154 = Unbundle By Name(w359) -> ("id"=w356:u16, "flowid"=w358:u16, "量程"=w357:u16, "工作状态"=w336:u16, "A"=→"A":sgl, "B"=→"B":sgl, "K"=→"K":sgl, "当前滴定数"=→"当前滴定数":sgl, "T"=→"环境温度":sgl, "H"=→"环境湿度":sgl, "运行时间"=→"运行时间":sgl, "当前ORP值"=→"ORP值":sgl, "加热实时温度"=→"加热实时温度":sgl, "当前步骤剩余时间"=→"当前步骤剩余时间":sgl, "结束滴定数"=→"终点滴定数":sgl, "注射泵保温温度"=→"注射泵保温温度":sgl, "匹配滴定数X0"=→"X0":u16)
    n155 = Unbundle By Name(w324) -> ("日志代码"=w341:u16)
    n156 = Unbundle By Name(w346) -> ("工作状态"=w329:u16, "id"=w328:u16)
    n157 = Unbundle By Name(w350) -> ("id"=w349:u16, "故障代码"=w307:u16, "告警代码"=w306:u16)
    n158 = Unbundle By Name(w344) -> ("日志代码"=w301:u16)
    n159 = local read "总步数"() -> (w300:i32)
    n160 = feedback-in #2(w341) -> ()
    n161 = feedback #2(w341) -> (w364:u16)
    n162 = feedback #3(w307) -> (w347:u16)
    n163 = feedback-in #3(w307) -> ()
    n164 = feedback #4(w306) -> (w323:u16)
    n165 = feedback-in #4(w306) -> ()
    n166 = Not Equal To 0?(x=w329) -> (x != 0?=w331:bool)
    n167 = Subtract(x=w341, y=1) -> (x-y=→"多列列表框":i32)
    n168 = Divide(x=w301, y=w300) -> (x/y=w303:dbl)
    n169 = Not Equal?(x=w341, y=w364) -> (x != y?=w363:bool)
    n170 = Not Equal?(x=w347, y=w307) -> (x != y?=w348:bool)
    n171 = Not Equal?(x=w323, y=w306) -> (x != y?=w322:bool)
    n172 = call <vilib>:"Boolean Crossing PtByPt.vi"("direction"=enum16{"either", "false-true", "true-false"}."false-true", "input"=w331) -> ("crossing"=w333:bool)  [unwired: 1 in]
    n173 = call <vilib>:"Boolean Crossing PtByPt.vi"("direction"=enum16{"either", "false-true", "true-false"}."true-false", "input"=w331) -> ("crossing"=w330:bool)  [unwired: 1 in]
    n174 = feedback #5(w301) -> (w345:u16)
    n175 = feedback-in #5(w301) -> ()
    n176 = Multiply(x=w303, y=100.0) -> (x*y=→"滑动杆":dbl)
    n177 = Not Equal?(x=w301, y=w345) -> (x != y?=w343:bool)
    n178 = property on="多列列表框" class="MCListbox (严格)"() -> ("ItemNames"=w319:string[][])  [unwired: 2 in, 2 out]
    n179 = case shown="真" w363 {
      tunnel: w341 -> [_ w518]
      frame False {
      }
      frame True {
        n180 = Subtract(x=w518, y=1) -> (x-y=w516:i32)
        n181 = Subtract(x=w516, y=5) -> (x-y=w520:i32)
        n182 = Greater Or Equal To 0?(x=w520) -> (x >= 0?=w519:bool)
        n183 = property on="多列列表框" class="MCListbox (严格)"() -> (error out=w524:errorcluster, "TopLeft"=w525:T21)  [unwired: 2 in, 1 out]
        n184 = Select(t=w520, s=w519, f=0) -> (s? t:f=w521:i32)
        n185 = Bundle By Name(cluster=w525, "Row"=w521) -> (w526:T21)
        n186 = property on="多列列表框" class="MCListbox (严格)"(error in=w524, "TopLeft"=w526) -> ()  [unwired: 1 in, 2 out]
      }
    }
    n187 = case shown="真" w333 {
      tunnel: w328 -> [_ w387]
      tunnel: w329 -> [_ w392]
      frame False {
      }
      frame True {
        n188 = case shown="8" w392 {
          tunnel: [_ "【水样测试】" ("字符串") "【标样核查】" ("字符串") "【零点核查】" ("字符串") "【跨度核查】" ("字符串") "【空白测试】" ("字符串") "【平行样测试】" ("字符串") "【加标回收】" ("字符串") "【空白校准】" ("字符串") "【标样校准】" ("字符串")] -> w391
          frame 0, Default {
          }
          frame 1 {
          }
          frame 2 {
          }
          frame 3 {
          }
          frame 4 {
          }
          frame 5 {
          }
          frame 6 {
          }
          frame 7 {
          }
          frame 8 {
          }
          frame 9 {
          }
        }
        n189 = call "id参数转换.vi"("id"=w387) -> ("table输出"=w386:string)  [unwired: 10 in]
        n190 = Concatenate Strings("<<" ("字符串"), w391, "启动" ("字符串")) -> (w390:string)
        n191 = Get Date/Time In Seconds() -> (seconds since 1Jan1904=w394:timestamp)
        n192 = Bundle By Name(cluster=T19 {"时间标识"=timestamp(0 s since 1904-01-01), "设备"="", "日志信息"="", "流程参数"=""} ("data in"), "时间标识"=w394, "设备"=w386, "日志信息"=w390) -> (w393:T19)
        n193 = call "CODMn操作日志.vi"("data in"=w393) -> ()  [unwired: 11 in]
      }
    }
    n194 = case shown="真" w330 {
      tunnel: w328 -> [_ w369]
      tunnel: w329 -> [_ w373]
      frame False {
      }
      frame True {
        n195 = case shown="1" w373 {
          tunnel: [_ "【水样测试】" ("字符串") "【标样核查】" ("字符串") "【零点核查】" ("字符串") "【跨度核查】" ("字符串") "【空白测试】" ("字符串") "【平行样测试】" ("字符串") "【加标回收】" ("字符串") "【空白校准】" ("字符串") "【标样校准】" ("字符串")] -> w372
          frame 0, Default {
          }
          frame 1 {
          }
          frame 2 {
          }
          frame 3 {
          }
          frame 4 {
          }
          frame 5 {
          }
          frame 6 {
          }
          frame 7 {
          }
          frame 8 {
          }
          frame 9 {
          }
        }
        n196 = call "id参数转换.vi"("id"=w369) -> ("table输出"=w368:string)  [unwired: 10 in]
        n197 = Concatenate Strings(w372, "停止" ("字符串"), ">>" ("字符串")) -> (w371:string)
        n198 = Get Date/Time In Seconds() -> (seconds since 1Jan1904=w375:timestamp)
        n199 = Bundle By Name(cluster=T19 {"时间标识"=timestamp(0 s since 1904-01-01), "设备"="", "日志信息"="", "流程参数"=""} ("data in"), "时间标识"=w375, "设备"=w368, "日志信息"=w371) -> (w374:T19)
        n200 = call "CODMn操作日志.vi"("data in"=w374) -> ()  [unwired: 11 in]
      }
    }
    n201 = case shown="0" w329 {
      frame 0 {
        n202 = local write "数组"(string[] [] ("数组")) -> ()
      }
      frame 1, Default {
      }
    }
    n203 = Not Equal To 0?(x=w336) -> (x != 0?=w361:bool)
    n204 = case shown="真" w343 {
      frame False {
      }
      frame True {
        n205 = property on="多列列表框" class="MCListbox (严格)"() -> ("ItemNames"=w409:string[][], "Value"=w410:i32)  [unwired: 2 in, 2 out]
        n206 = Index Array(array=w409, index (row)=w410) -> (element=w408:string[])  [unwired: 1 in]
        n207 = Index Array(array=w408) -> (element=w407:string)  [unwired: 1 in]
        n208 = call "过滤筛选流程.vi"("字符串"=w407) -> ("匹配后偏移量"=w406:i32)  [unwired: 10 in]
        n209 = case shown="默认" w406 {
          tunnel: w407 -> [_ w411]
          frame -1 {
          }
          frame Default {
            # "步骤日志存储"
            n210 = case shown="默认" w411 {
              selector: w411 -> [w417 w419]
              tunnel: [w417 w419] -> w413
              tunnel: [string[] [] ("数组") "数组"] -> w412
              frame "读数" {
              }
              frame Default {
              }
            }
            n211 = for {
              N: 1 -> [_]
              tunnel: w413 -> [w421]
              shift-right: [w420] -> w414
              shift-left: w412 -> [w422]
              n212 = Search 1D Array(1D array=w422, element=w421) -> (index of element=w425:i32)  [unwired: 1 in]
              n213 = Format Into String(format string="%s" ("格式字符串"), w421) -> (resulting string=w426:string)  [unwired: 2 in, 1 out]
              n214 = Equal?(x=w425, y=-1) -> (x = y?=w423:bool)
              n215 = case shown="真" w423 {
                tunnel: w426 -> [_ w434]
                tunnel: w422 -> [w428 w438]
                tunnel: w421 -> [_ w437]
                tunnel: [w428 w436] -> w420
                frame False {
                }
                frame True {
                  n216 = Insert Into Array(array=w438, new element=w437) -> (w436:string[])  [unwired: 1 in]
                  n217 = case shown="\"初始化\"" w434 {
                    selector: w434 -> [w463 w466 w469]
                    tunnel: [w463 w465 w468] -> w430
                    frame Default {
                    }
                    frame "初始化" {
                      n218 = Concatenate Strings("<<" ("字符串"), w466) -> (w465:string)
                    }
                    frame "结束" {
                      n219 = Concatenate Strings(w469, ">>" ("字符串")) -> (w468:string)
                    }
                  }
                  n220 = global read "VARCODMn全局变量.vi" "状态告警区"() -> (w433:T17)
                  n221 = Unbundle By Name(w433) -> ("工作状态"=w432:u16)
                  n222 = global read "VARCODMn全局变量.vi" "状态告警区"() -> (w453:T17)
                  n223 = case shown="1" w432 {
                    tunnel: [_ "【水样测试】" ("字符串") "【标样核查】" ("字符串") "【零点核查】" ("字符串") "【跨度核查】" ("字符串") "【空白测试】" ("字符串") "【平行样测试】" ("字符串") "【加标回收】" ("字符串") "【空白校准】" ("字符串") "【标样校准】" ("字符串")] -> w431
                    frame 0, Default {
                    }
                    frame 1 {
                    }
                    frame 2 {
                    }
                    frame 3 {
                    }
                    frame 4 {
                    }
                    frame 5 {
                    }
                    frame 6 {
                    }
                    frame 7 {
                    }
                    frame 8 {
                    }
                    frame 9 {
                    }
                  }
                  n224 = global read "VARCODMn全局变量.vi" "状态告警区"() -> (w448:T17)
                  n225 = Unbundle By Name(w453) -> ("id"=w452:u16)
                  n226 = case shown="1, 21, 131" w452 {
                    tunnel: [_ "CODMn" ("table输入") "氨氮" ("table输入") "总氮" ("table输入")] -> w450
                    frame Default {
                    }
                    frame 1, 21, 131 {
                    }
                    frame 3, 92 {
                    }
                    frame 2, 76 {
                    }
                  }
                  n227 = Unbundle By Name(w448) -> ("A"=w445:sgl, "B"=w444:sgl, "K"=w443:sgl, "当前滴定数"=w442:sgl, "id"=w441:u16, "flowid"=w440:u16, "量程"=w439:u16)
                  n228 = Concatenate Strings(w431, w430) -> (w429:string)
                  n229 = Format Into String(format string="A=%#f,B=%#f,K=%#f,当前滴定数=%#f,Flow=%d-%-d-%-d" ("格式字符串"), w445, w444, w443, w442, w441, w440, w439) -> (resulting string=w446:string)  [unwired: 2 in, 1 out]
                  n230 = Get Date/Time In Seconds() -> (seconds since 1Jan1904=w449:timestamp)
                  n231 = Bundle By Name(cluster=T19 {"时间标识"=timestamp(0 s since 1904-01-01), "设备"="", "日志信息"="", "流程参数"=""} ("data in"), "时间标识"=w449, "设备"=w450, "日志信息"=w429, "流程参数"=w446) -> (w451:T19)
                  n232 = call "CODMn操作日志.vi"("data in"=w451) -> ()  [unwired: 11 in]
                }
              }
            }
            n233 = local write "数组"(w414) -> ()
          }
        }
      }
    }
    n234 = Not Equal To 0?(x=w306) -> (x != 0?=w308:bool)
    n235 = Not Equal To 0?(x=w307) -> (x != 0?=w309:bool)
    n236 = call <vilib>:"Boolean Crossing PtByPt.vi"("direction"=enum16{"either", "false-true", "true-false"}."either", "input"=w361) -> ("crossing"=w335:bool)  [unwired: 1 in]
    n237 = Or(x=w309, y=w308) -> (x .or. y?=w305:bool)
    n238 = Empty Array?(array=w319) -> (empty?=w318:bool)
    n239 = Bundle("id"=w356, "flowid"=w358, "量程"=w357) -> (w351:cluster{"id":u16, "flowid":u16, "量程":u16})  [unwired: 1 in]
    n240 = First Call?() -> (First Call?: T/F=w362:bool)
    n241 = Compound Arithmetic op=OR ("复合运算")(w335, w362, w318) -> (w360:bool)
    n242 = while {
      tunnel: w360 -> [w504]
      tunnel: w351 -> [w503]
      shift-right: [w500] -> _
      shift-left: _ -> [w501]
      shift-right: [w497] -> _
      shift-left: _ -> [w499]
      stop <- TRUE stop-if-true
      # "XML解析步骤显示"
      n243 = case shown="真" w504 {
        tunnel: [w506 w514] -> w497
        tunnel: [w505 w513] -> w500
        tunnel: w503 -> [_ w508]
        tunnel: w499 -> [w506 _]
        tunnel: w501 -> [w505 _]
        frame False {
        }
        frame True {
          n244 = call "斯坦道XML解析.vi"("添加的路径"="流程路径", "参数簇"=w508) -> ("步骤时间"=w509:string[], "步骤名"=w511:string[])  [unwired: 8 in]
          n245 = for {
            tunnel: w511 -> [_] mode=indexing
            tunnel: [w515] -> w512 mode=indexing
            i -> [w515]
          }
          n246 = Build Array(w511, w509) -> (w510:string[][])
          n247 = Transpose 2D Array(2D array=w510) -> (transposed array=w513:string[][])
          n248 = Number To Decimal String(number=w512) -> (decimal integer string=w514:string[])  [unwired: 1 in]
        }
      }
      n249 = Array Size(array=w497) -> (size(s)=→"总步数":i32)
      n250 = property on="多列列表框" class="MCListbox (严格)"("ItemNames"=w500, "RowHdrs[]"=w497) -> ()  [unwired: 2 in, 2 out]
    }
    n251 = case shown="真" w305 {
      tunnel: w349 -> [_ w479]
      tunnel: w348 -> [_ w478]
      tunnel: w322 -> [_ w476]
      tunnel: w306 -> [_ w475]
      tunnel: w321 -> [_ w474]
      tunnel: w307 -> [_ w473]
      frame False {
      }
      frame True {
        n252 = Or(x=w476, y=w478) -> (x .or. y?=w477:bool)
        n253 = case shown="真" w477 {
          tunnel: w479 -> [_ w494]
          tunnel: w473 -> [_ w486]
          tunnel: w475 -> [_ w485]
          tunnel: w474 -> [_ w484]
          frame False {
          }
          frame True {
            n254 = call "故障码字段定义.vi"("故障代码"=w486) -> ("字符串"=w482:string)  [unwired: 10 in]
            n255 = call "告警码字段定义.vi"("告警代码"=w485) -> ("故障详情"=w480:string, "通用告警信息"=w481:string)  [unwired: 8 in, 1 out]
            n256 = Format Into String(format string="【%s】%s" ("格式字符串"), initial string="" ("初始字符串"), w482, w481) -> (resulting string=w491:string)  [unwired: 1 in, 1 out]
            n257 = call "id参数转换.vi"("id"=w494) -> ("table输出"=w483:string)  [unwired: 10 in]
            n258 = Search and Replace String(replace all?=TRUE ("替换全部？(F)"), input string=w491, search string="【无故障】|无告警" ("字符串")) -> (result string=w488:string)  [unwired: 5 in, 3 out]
            n259 = call "balloon入队列.vi"("队列"=w484, "故障详情"=w480, "告警信息"=w481, "故障信息"=w482, "参数名称"=w483) -> ()  [unwired: 6 in, 1 out]
            n260 = Get Date/Time In Seconds() -> (seconds since 1Jan1904=w495:timestamp)
            n261 = Bundle By Name(cluster=T20 {"时间标识"=timestamp(0 s since 1904-01-01), "设备"="", "日志信息"="", "备注"=""} ("data in"), "时间标识"=w495, "设备"=w483, "日志信息"=w488, "备注"=w480) -> (w496:T20)
            n262 = call "CODMn报警信息.vi"("data in"=w496) -> ()  [unwired: 10 in, 1 out]
          }
        }
      }
    }
    n263 = global read "VARCODMn全局变量.vi" "ORP滴定曲线"() -> (→"ORP滴定曲线":u16[])
    n264 = global read "VARCODMn全局变量.vi" "滴定数-ORP值"() -> (→"滴定数-ORP值":u16[])
    n265 = global read "VARCODMn全局变量.vi" "波形时间"() -> (→"波形时间":timestamp)
    n266 = global read "VARCODMn全局变量.vi" "温度波形时间"() -> (→"温度波形时间":timestamp)
    n267 = global read "VARCODMn全局变量.vi" "时间-温度"() -> (→"时间-温度":u16[])
    n268 = global read "VARCODMn全局变量.vi" "温度曲线"() -> (→"ORP滴定曲线 2":u16[])
  }
  n269 = control-ref of="测量模式下拉列表"() -> (w52:refnum<vi>)
  n270 = control-ref of="校准按钮"() -> (w22:refnum<vi>)
  n271 = control-ref of="参数下拉列表"() -> (w53:refnum<vi>)
  n272 = control-ref of="量程下拉列表"() -> (w54:refnum<vi>)
  n273 = control-ref of="校准按钮"() -> (w43:refnum<vi>)
  n274 = control-ref of="曲线模型"() -> (w42:refnum<vi>)
  n275 = control-ref of="公式"() -> (w51:refnum<vi>)
  n276 = while {
    tunnel: w44 -> [w530]
    tunnel: w22 -> [w528]
    tunnel: w21 -> [w527]
    tunnel: w18 -> [_]
    tunnel: w10 -> [_]
    stop <- FALSE stop-if-true
    n277 = event shown="[3] \"曲线模型.标液浓度1\", \"曲线模型.测量吸光度1\", \"曲线模型.标液浓度2\", \"曲线模型.测量吸光度2\", \"曲线模型.样品1启用\", \"曲线模型.样品2启用\", \"曲线模型.标液浓度3\", \"曲线模型.测量吸光度3\", \"曲线模型.样品3启用\", \"曲线模型.标液浓度4\", \"曲线模型.测量吸光度4\", \"曲线模型.样品4启用\", \"曲线模型.标液浓度5\", \"曲线模型.测量吸光度5\", \"曲线模型.样品5启用\", \"曲线模型.模型\", \"曲线模型.method\", \"曲线模型.精度\": 值改变" {
      selector: _ -> [_ _ _ _ _ _ _]
      dyn-events: _ -> [_ _ _ _ _ _ _]
      timeout: _ -> [_ _ _ _ _ _ _]
      tunnel: [_ _ _ w555 w612 w775 w817] -> w529
      tunnel: w527 -> [_ _ _ w554 w615 w786 w813]
      tunnel: w528 -> [_ _ _ _ w614 w790 _]
      tunnel: w530 -> [_ _ _ _ w613 _ _]
      event Timeout {
        # "始终在超时后终止\n事件结构。在事件结构的其它情况下决不终止循环。"
        n278 = event-data() -> ()  [unwired: 1 in, 2 out]
      }
      event "曲线模型.标液浓度1", "曲线模型.标液浓度2", "曲线模型.标液浓度3", "曲线模型.标液浓度4", "曲线模型.标液浓度5", "曲线模型.精度": Mouse Down {
        n279 = event-data() -> ("CtlRef"=w536:refnum<vi>)  [unwired: 1 in, 7 out]
        n280 = property class="DigNum (严格)"(reference=w536) -> (reference out=w535:refnum<vi>, "Value"=w532:dbl)  [unwired: 1 in, 1 out]
        n281 = call "数字键盘.vi"("OldNumber"=w532) -> ("NewNumber"=w533:dbl)
        n282 = Equal?(x=w532, y=w533) -> (x = y?=w534:bool)
        n283 = case shown="假" w534 {
          tunnel: w535 -> [w538 _]
          tunnel: w533 -> [w537 _]
          frame False {
            n284 = property class="DigNum (严格)"(reference=w538, "Val(Sgnl)"=w537) -> ()  [unwired: 1 in, 2 out]
          }
          frame True {
          }
        }
      }
      event "曲线模型.测量吸光度1", "曲线模型.测量吸光度2", "曲线模型.测量吸光度3", "曲线模型.测量吸光度4", "曲线模型.测量吸光度5": Mouse Down {
        n285 = event-data() -> ("CtlRef"=w542:refnum<vi>)  [unwired: 1 in, 7 out]
        n286 = property class="DigNum (严格)"(reference=w542) -> (reference out=w541:refnum<vi>, "Value"=w540:dbl)  [unwired: 1 in, 1 out]
        n287 = call "数字键盘.vi"("OldNumber"=w540) -> ("NewNumber"=w539:dbl)
        n288 = property class="DigNum (严格)"(reference=w541, "Val(Sgnl)"=w539) -> ()  [unwired: 1 in, 2 out]
      }
      event "曲线模型.标液浓度1", "曲线模型.测量吸光度1", "曲线模型.标液浓度2", "曲线模型.测量吸光度2", "曲线模型.样品1启用", "曲线模型.样品2启用", "曲线模型.标液浓度3", "曲线模型.测量吸光度3", "曲线模型.样品3启用", "曲线模型.标液浓度4", "曲线模型.测量吸光度4", "曲线模型.样品4启用", "曲线模型.标液浓度5", "曲线模型.测量吸光度5", "曲线模型.样品5启用", "曲线模型.模型", "曲线模型.method", "曲线模型.精度": Value Change {
        n289 = event-data() -> ()  [unwired: 1 in, 6 out]
        n290 = property class="Clust (严格)"(reference=w554) -> ("Value"=w553:T5)  [unwired: 1 in, 2 out]
        n291 = call <vilib>:"Application Directory.vi"() -> ("Application Directory"=w574:path)
        n292 = Build Path(base path=w574, name or relative path="config" ("名称或相对路径")) -> (appended path=w572:path)
        n293 = Unbundle By Name(w553) -> ("模型"=w598:enum32{"线性", "多项式"}, "标液浓度1"=w594:dbl, "标液浓度2"=w593:dbl, "标液浓度3"=w592:dbl, "标液浓度4"=w591:dbl, "标液浓度5"=w590:dbl, "测量吸光度1"=w587:dbl, "测量吸光度2"=w586:dbl, "测量吸光度3"=w585:dbl, "测量吸光度4"=w584:dbl, "测量吸光度5"=w583:dbl, "样品1启用"=w581:bool, "样品2启用"=w580:bool, "样品3启用"=w579:bool, "样品4启用"=w578:bool, "样品5启用"=w577:bool, "method"=w597:enum16{"最小二乘", "最小绝对残差", "Bisquare"}, "精度"=w596:dbl)
        n294 = call <vilib>:"Check if File or Folder Exists.vi"("path"=w572) -> ("file or folder exists?"=w571:bool, "dup path"=w570:path)  [unwired: 8 in, 1 out]
        n295 = case shown="真" w571 {
          tunnel: w570 -> [w608 w609]
          tunnel: [w607 w609] -> w567
          frame False {
            n296 = Create Folder(path (use dialog)=w608) -> (created path=w607:path)  [unwired: 2 in, 2 out]
          }
          frame True {
          }
        }
        n297 = Insert Into Array(array=dbl[] [] ("标液浓度"), new element #1=w594, new element #2=w593, new element #3=w592, new element #4=w591, new element #5=w590) -> (w589:dbl[])  [unwired: 1 in]
        n298 = Insert Into Array(array=dbl[] [] ("标液浓度"), new element #1=w587, new element #2=w586, new element #3=w585, new element #4=w584, new element #5=w583) -> (w546:dbl[])  [unwired: 1 in]
        n299 = Insert Into Array(array=bool[] [] ("启用"), new element #1=w581, new element #2=w580, new element #3=w579, new element #4=w578, new element #5=w577) -> (w547:bool[])  [unwired: 1 in]
        n300 = for {
          tunnel: w547 -> [w602] mode=indexing
          tunnel: w546 -> [w601] mode=indexing
          shift-right: [w599] -> w544
          shift-left: dbl[] [] -> [w600]
          n301 = case shown="真" w602 {
            tunnel: w601 -> [_ w606]
            tunnel: w600 -> [w603 w605]
            tunnel: [w603 w604] -> w599
            frame False {
            }
            frame True {
              n302 = Build Array (concatenate)(w605, w606) -> (w604:dbl[])
            }
          }
        }
        n303 = Concatenate Strings("曲线模型" ("字符串"), ".ini" ("字符串")) -> (w569:string)
        n304 = call "CODMn线性公式.vi"("标液浓度"=w589, "监测浓度"=w546, "启用"=w547, "method"=w597, "模型"=w598, "精度"=w596) -> ("拟合方程"=w576:string, "r^2"=w550:dbl, "XY图"=w575:cluster{"X Values":dbl[], "Y Values":dbl[]}[], "Polynomial Coefficients"=w551:dbl[])  [unwired: 7 in, 3 out]
        n305 = Bundle By Name(cluster=w553, "拟合公式"=w576, "r^2"=w550, "XY图"=w575) -> (w552:T5)
        n306 = local write "曲线模型"(w552) -> ()
        n307 = Array Max & Min(array=w544) -> (max value=w543:dbl)  [unwired: 3 out]
        n308 = Bundle By Name(cluster=T10 {"曲线模型"={"标液浓度1"=0.0, "测量吸光度1"=0.0, "样品1启用"=FALSE, "标液浓度2"=0.0, "测量吸光度2"=0.0, "样品2启用"=FALSE, "标液浓度3"=0.0, "测量吸光度3"=0.0, "样品3启用"=FALSE, "标液浓度4"=0.0, "测量吸光度4"=0.0, "样品4启用"=FALSE, "标液浓度5"=0.0, "测量吸光度5"=0.0, "样品5启用"=FALSE, "模型"=enum."线性", "method"=enum."最小二乘", "精度"=7.0, "XY图"=[], "拟合公式"="", "r^2"=0.0, "零点校准时间"=timestamp(0 s since 1904-01-01), "标液校准时间1"=timestamp(0 s since 1904-01-01), "标液校准时间2"=timestamp(0 s since 1904-01-01), "标液校准时间3"=timestamp(0 s since 1904-01-01), "标液校准时间4"=timestamp(0 s since 1904-01-01)}, "Polynomial Coefficients"=[]} ("输出簇"), "曲线模型"=w552, "Polynomial Coefficients"=w551) -> (w559:T10)
        n309 = Build Path(base path=w567, name or relative path=w569) -> (appended path=w560:path)
        n310 = Array To Cluster(array=w551) -> (cluster=w549:T15)
        n311 = local read "模型选择"() -> (w558:cluster{"参数":u8, "测量模式":u8, "量程":u8})
        n312 = local write "公式切换阈值滴定数(0~9999)"(w543) -> ()
        n313 = local write "公式"(w549) -> ()
        n314 = Flatten To String(anything=w558) -> (data string=w566:string)  [unwired: 3 in, 2 out]
        n315 = call <vilib>:"Open Config Data.vi"("configuration file path"=w560) -> ("error out"=w563:errorcluster, "refnum"=w564:T12)  [unwired: 8 in, 1 out]
        n316 = local read "公式、校准输出"() -> (w557:T6)
        n317 = call <userlib>:"Write Section Cluster__ogtk.vi"("section (optional)"=w566, "error in (no error)"=w563, "Section Formatted Cluster"=w559, "refnum"=w564) -> ("error out"=w561:errorcluster, "dup refnum"=w562:T12)  [unwired: 6 in]
        n318 = Bundle By Name(cluster=w557, "公式"=w549, "校准.校准？"=FALSE) -> (w555:T6)
        n319 = call <vilib>:"Close Config Data.vi"("error in (no error)"=w561, "refnum"=w562) -> ()  [unwired: 8 in, 2 out]
        n320 = global write "CODMn断电保存全局变量.vi" "公式、校准输出"(w555) -> ()
      }
      event "校准按钮.校准1", "校准按钮.校准2", "校准按钮.校准3", "校准按钮.校准4", "校准按钮.校准5": Mouse Down {
        n321 = event-data() -> ("CtlRef"=w616:refnum<vi>)  [unwired: 1 in, 7 out]
        n322 = property class="Bool (严格)"(reference=w616) -> ("Label.Text"=w611:string)  [unwired: 1 in, 2 out]
        n323 = case shown="\"校准1\"" w611 {
          tunnel: [FALSE ("T button?") w618 w622 w626 w630 w634] -> w610
          frame "假", Default {
          }
          frame "校准1" {
            n324 = Two Button Dialog(message="是否选择数据表中已有的空白校准数据" ("消息"), 1:"否" ("F按钮名称（“取消”）"), 2:"是" ("T按钮名称（“确定”）")) -> (T button?=w618:bool)
          }
          frame "校准2" {
            n325 = Two Button Dialog(message="是否选择数据表中已有的标样校准数据" ("消息"), 1:"否" ("F按钮名称（“取消”）"), 2:"是" ("T按钮名称（“确定”）")) -> (T button?=w622:bool)
          }
          frame "校准3" {
            n326 = Two Button Dialog(message="是否选择数据表中已有的标样核查数据" ("消息"), 1:"否" ("F按钮名称（“取消”）"), 2:"是" ("T按钮名称（“确定”）")) -> (T button?=w626:bool)
          }
          frame "校准4" {
            n327 = Two Button Dialog(message="是否选择数据表中已有的零点核查数据" ("消息"), 1:"否" ("F按钮名称（“取消”）"), 2:"是" ("T按钮名称（“确定”）")) -> (T button?=w630:bool)
          }
          frame "校准5" {
            n328 = Two Button Dialog(message="是否选择数据表中已有的跨度核查数据" ("消息"), 1:"否" ("F按钮名称（“取消”）"), 2:"是" ("T按钮名称（“确定”）")) -> (T button?=w634:bool)
          }
        }
        n329 = case shown="真" w610 {
          tunnel: w611 -> [w650 w682]
          tunnel: w615 -> [w646 w681]
          tunnel: w614 -> [w645 _]
          tunnel: w613 -> [w641 _]
          tunnel: [w640 w683] -> w612
          frame False {
            w644 = T22."Disabled and Grayed Out" ("禁用")
            n330 = case shown="\"校准5\"" w650 {
              tunnel: [w672 w673 w676 w677 w679] -> w648
              tunnel: [u16 1 ("校准点1-5") u16 2 ("校准点1-5") u16 3 ("校准点1-5") u16 4 ("校准点1-5") u16 5 ("校准点1-5")] -> w638
              frame "校准1", Default {
                n331 = control-ref of="标液浓度1"() -> (w672:refnum<vi>)
              }
              frame "校准2" {
                n332 = control-ref of="标液浓度2"() -> (w673:refnum<vi>)
              }
              frame "校准3" {
                n333 = control-ref of="标液浓度3"() -> (w676:refnum<vi>)
              }
              frame "校准4" {
                n334 = control-ref of="标液浓度4"() -> (w677:refnum<vi>)
              }
              frame "校准5" {
                n335 = control-ref of="标液浓度5"() -> (w679:refnum<vi>)
              }
            }
            n336 = property class="DigNum (严格)"(reference=w648) -> ("Value"=w643:dbl)  [unwired: 1 in, 2 out]
            n337 = local read "量程下拉列表"() -> (w639:enum16{"低量程1", "低量程2", "高量程1", "高量程2"})
            n338 = property class="Clust (严格)"(reference=w645, "DisabledEnum"=w644) -> ()  [unwired: 1 in, 2 out]
            n339 = property class="Clust (严格)"(reference=w646, "DisabledEnum"=w644) -> ()  [unwired: 1 in, 2 out]
            n340 = Equal To 0?(x=w643) -> ()  [unwired: 1 out]
            n341 = case shown="1" w638 {
              tunnel: [w651 w655 w659 w663 w668] -> w642
              tunnel: w639 -> [w652 w656 w660 w664 w667]
              frame 2, Default {
                # "校标"
                n342 = case shown="\"高量程1\"" w652 {
                  tunnel: [cluster{"命令":string, "data":variant} {"命令"="启动", "data"=variant(cluster{"站号":u16, "控制命令":u16[]} {"站号"=21, "控制命令"=[2304, 0]})} ("元素") cluster{"命令":string, "data":variant} {"命令"="启动", "data"=variant(cluster{"站号":u16, "控制命令":u16[]} {"站号"=21, "控制命令"=[2304, 256]})} ("元素")] -> w651
                  frame "低量程1", Default {
                  }
                  frame "高量程1" {
                  }
                }
              }
              frame 3 {
                # "标样核查"
                n343 = case shown="\"低量程1\", 默认" w656 {
                  tunnel: [w657 cluster{"命令":string, "data":variant} {"命令"="启动", "data"=variant(cluster{"站号":u16, "控制命令":u16[]} {"站号"=21, "控制命令"=[512, 256]})} ("元素")] -> w655
                  frame "低量程1", Default {
                    w657 = cluster{"命令":string, "data":variant} {"命令"="启动", "data"=variant(cluster{"站号":u16, "控制命令":u16[]} {"站号"=21, "控制命令"=[512, 0]})}  # 标样核查
                  }
                  frame "高量程1" {
                  }
                }
              }
              frame 4 {
                # "零点核查"
                n344 = case shown="\"高量程1\"" w660 {
                  tunnel: [w661 cluster{"命令":string, "data":variant} {"命令"="启动", "data"=variant(cluster{"站号":u16, "控制命令":u16[]} {"站号"=21, "控制命令"=[768, 256]})} ("元素")] -> w659
                  frame "低量程1", Default {
                    w661 = cluster{"命令":string, "data":variant} {"命令"="启动", "data"=variant(cluster{"站号":u16, "控制命令":u16[]} {"站号"=21, "控制命令"=[768, 0]})}  # 零点核查
                  }
                  frame "高量程1" {
                  }
                }
              }
              frame 5 {
                # "跨度核查"
                n345 = case shown="\"低量程1\", 默认" w664 {
                  tunnel: [w665 cluster{"命令":string, "data":variant} {"命令"="启动", "data"=variant(cluster{"站号":u16, "控制命令":u16[]} {"站号"=21, "控制命令"=[1024, 256]})} ("元素")] -> w663
                  frame "低量程1", Default {
                    w665 = cluster{"命令":string, "data":variant} {"命令"="启动", "data"=variant(cluster{"站号":u16, "控制命令":u16[]} {"站号"=21, "控制命令"=[1024, 0]})}  # 跨度核查
                  }
                  frame "高量程1" {
                  }
                }
              }
              frame 1 {
                # "校零"
                n346 = case shown="\"高量程1\"" w667 {
                  tunnel: [cluster{"命令":string, "data":variant} {"命令"="启动", "data"=variant(cluster{"站号":u16, "控制命令":u16[]} {"站号"=21, "控制命令"=[2048, 0]})} ("元素") cluster{"命令":string, "data":variant} {"命令"="启动", "data"=variant(cluster{"站号":u16, "控制命令":u16[]} {"站号"=21, "控制命令"=[2048, 256]})} ("元素")] -> w668
                  frame "低量程1", Default {
                  }
                  frame "高量程1" {
                  }
                }
              }
            }
            n347 = local read "公式、校准输出"() -> (w647:T6)
            n348 = Bundle By Name(cluster=w647, "校准.校准？"=TRUE ("校准？"), "校准.校准点1-5"=w638, "校准.校准浓度"=w643) -> (w640:T6)
            n349 = global write "CODMn断电保存全局变量.vi" "公式、校准输出"(w640) -> ()
            n350 = Enqueue Element(queue=w641, element=w642) -> ()  [unwired: 2 in, 3 out]
          }
          frame True {
            n351 = case shown="\"校准2\"" w682 {
              tunnel: w681 -> [_ w688 w706 w724 w742 w760]
              frame "假", Default {
              }
              frame "校准1" {
                n352 = property class="Clust (严格)"(reference=w688) -> ("Value"=w687:T5)  [unwired: 1 in, 2 out]
                n353 = call "校准数据选择表.vi"("condition"="where 测量模式=\"空白校准\" and 数据标识 =\"N\" order by 时间 desc") -> ("布尔"=w684:bool, "ItemNames"=w686:string[])  [unwired: 9 in]
                n354 = case shown="真" w684 {
                  tunnel: w688 -> [_ w701]
                  tunnel: w687 -> [_ w700]
                  tunnel: w686 -> [_ w695]
                  frame False {
                  }
                  frame True {
                    n355 = Index Array(array=w695, index #2=7 ("索引"), index #3=11 ("索引")) -> (element #1=w692:string, element #2=w690:string, element #3=w691:string)  [unwired: 1 in]
                    n356 = Scan From String(format string="%<%Y/%m/%d %H:%M:%S>T" ("格式字符串"), input string=w692) -> (output 1=w697:timestamp)  [unwired: 3 in, 3 out]
                    n357 = Fract/Exp String To Number(string=w690) -> (number=w689:dbl)  [unwired: 3 in, 1 out]
                    n358 = Decimal String To Number(string=w691) -> (number=w696:i32)  [unwired: 2 in, 1 out]
                    n359 = Bundle By Name(cluster=w700, "标液浓度1"=w689, "测量吸光度1"=w696, "零点校准时间"=w697) -> (w699:T5)
                    n360 = property class="Clust (严格)"(reference=w701, "Val(Sgnl)"=w699) -> ()  [unwired: 1 in, 2 out]
                  }
                }
              }
              frame "校准2" {
                n361 = property class="Clust (严格)"(reference=w706) -> ("Value"=w705:T5)  [unwired: 1 in, 2 out]
                n362 = call "校准数据选择表.vi"("condition"="where 测量模式=\"标样校准\" and 数据标识 =\"N\" order by 时间 desc") -> ("布尔"=w702:bool, "ItemNames"=w704:string[])  [unwired: 9 in]
                n363 = case shown="真" w702 {
                  tunnel: w706 -> [_ w719]
                  tunnel: w705 -> [_ w718]
                  tunnel: w704 -> [_ w713]
                  frame False {
                  }
                  frame True {
                    n364 = Index Array(array=w713, index #2=7 ("索引"), index #3=11 ("索引")) -> (element #1=w710:string, element #2=w708:string, element #3=w709:string)  [unwired: 1 in]
                    n365 = Scan From String(format string="%<%Y/%m/%d %H:%M:%S>T" ("格式字符串"), input string=w710) -> (output 1=w715:timestamp)  [unwired: 3 in, 3 out]
                    n366 = Fract/Exp String To Number(string=w708) -> (number=w707:dbl)  [unwired: 3 in, 1 out]
                    n367 = Decimal String To Number(string=w709) -> (number=w714:i32)  [unwired: 2 in, 1 out]
                    n368 = Bundle By Name(cluster=w718, "标液浓度2"=w707, "测量吸光度2"=w714, "标液校准时间1"=w715) -> (w717:T5)
                    n369 = property class="Clust (严格)"(reference=w719, "Val(Sgnl)"=w717) -> ()  [unwired: 1 in, 2 out]
                  }
                }
              }
              frame "校准3" {
                n370 = property class="Clust (严格)"(reference=w724) -> ("Value"=w723:T5)  [unwired: 1 in, 2 out]
                n371 = call "校准数据选择表.vi"("condition"="where 测量模式=\"标样核查\" and 数据标识 =\"N\" order by 时间 desc") -> ("布尔"=w720:bool, "ItemNames"=w721:string[])  [unwired: 9 in]
                n372 = case shown="真" w720 {
                  tunnel: w724 -> [_ w737]
                  tunnel: w723 -> [_ w736]
                  tunnel: w721 -> [_ w728]
                  frame False {
                  }
                  frame True {
                    n373 = Index Array(array=w728, index #2=7 ("索引"), index #3=11 ("索引")) -> (element #1=w727:string, element #2=w726:string, element #3=w725:string)  [unwired: 1 in]
                    n374 = Scan From String(format string="%<%Y/%m/%d %H:%M:%S>T" ("格式字符串"), input string=w727) -> (output 1=w733:timestamp)  [unwired: 3 in, 3 out]
                    n375 = Fract/Exp String To Number(string=w726) -> (number=w732:dbl)  [unwired: 3 in, 1 out]
                    n376 = Decimal String To Number(string=w725) -> (number=w731:i32)  [unwired: 2 in, 1 out]
                    n377 = Bundle By Name(cluster=w736, "标液浓度3"=w732, "测量吸光度3"=w731, "标液校准时间2"=w733) -> (w735:T5)
                    n378 = property class="Clust (严格)"(reference=w737, "Val(Sgnl)"=w735) -> ()  [unwired: 1 in, 2 out]
                  }
                }
              }
              frame "校准4" {
                n379 = property class="Clust (严格)"(reference=w742) -> ("Value"=w741:T5)  [unwired: 1 in, 2 out]
                n380 = call "校准数据选择表.vi"("condition"="where 测量模式=\"零点核查\" and 数据标识 =\"N\" order by 时间 desc") -> ("布尔"=w738:bool, "ItemNames"=w739:string[])  [unwired: 9 in]
                n381 = case shown="真" w738 {
                  tunnel: w742 -> [_ w755]
                  tunnel: w741 -> [_ w754]
                  tunnel: w739 -> [_ w747]
                  frame False {
                  }
                  frame True {
                    n382 = Index Array(array=w747, index #2=7 ("索引"), index #3=11 ("索引")) -> (element #1=w746:string, element #2=w744:string, element #3=w745:string)  [unwired: 1 in]
                    n383 = Scan From String(format string="%<%Y/%m/%d %H:%M:%S>T" ("格式字符串"), input string=w746) -> (output 1=w751:timestamp)  [unwired: 3 in, 3 out]
                    n384 = Fract/Exp String To Number(string=w744) -> (number=w743:dbl)  [unwired: 3 in, 1 out]
                    n385 = Decimal String To Number(string=w745) -> (number=w750:i32)  [unwired: 2 in, 1 out]
                    n386 = Bundle By Name(cluster=w754, "标液浓度4"=w743, "测量吸光度4"=w750, "标液校准时间3"=w751) -> (w753:T5)
                    n387 = property class="Clust (严格)"(reference=w755, "Val(Sgnl)"=w753) -> ()  [unwired: 1 in, 2 out]
                  }
                }
              }
              frame "校准5" {
                n388 = property class="Clust (严格)"(reference=w760) -> ("Value"=w759:T5)  [unwired: 1 in, 2 out]
                n389 = call "校准数据选择表.vi"("condition"="where 测量模式=\"跨度核查\" and 数据标识 =\"N\" order by 时间 desc") -> ("布尔"=w756:bool, "ItemNames"=w757:string[])  [unwired: 9 in]
                n390 = case shown="真" w756 {
                  tunnel: w760 -> [_ w773]
                  tunnel: w759 -> [_ w772]
                  tunnel: w757 -> [_ w767]
                  frame False {
                  }
                  frame True {
                    n391 = Index Array(array=w767, index #2=7 ("索引"), index #3=11 ("索引")) -> (element #1=w766:string, element #2=w762:string, element #3=w763:string)  [unwired: 1 in]
                    n392 = Scan From String(format string="%<%Y/%m/%d %H:%M:%S>T" ("格式字符串"), input string=w766) -> (output 1=w769:timestamp)  [unwired: 3 in, 3 out]
                    n393 = Fract/Exp String To Number(string=w762) -> (number=w761:dbl)  [unwired: 3 in, 1 out]
                    n394 = Decimal String To Number(string=w763) -> (number=w768:i32)  [unwired: 2 in, 1 out]
                    n395 = Bundle By Name(cluster=w772, "标液浓度5"=w761, "测量吸光度5"=w768, "标液校准时间4"=w769) -> (w771:T5)
                    n396 = property class="Clust (严格)"(reference=w773, "Val(Sgnl)"=w771) -> ()  [unwired: 1 in, 2 out]
                  }
                }
              }
            }
            n397 = local read "公式、校准输出"() -> (w683:T6)
          }
        }
      }
      event "校准完毕": Value Change {
        w789 = T22."Enabled" ("禁用")
        n398 = event-data() -> ()  [unwired: 1 in, 6 out]
        n399 = local read "公式、校准输出"() -> (w788:T6)
        n400 = property class="Clust (严格)"(reference=w786) -> (reference out=w784:refnum<vi>, error out=w783:errorcluster, "Value"=w785:T5)  [unwired: 1 in]
        n401 = Unbundle By Name(w788) -> ("校准.校准点1-5"=w787:u16)
        n402 = global read "VARCODMn全局变量.vi" "状态告警区"() -> (w781:T17)
        n403 = property class="Clust (严格)"(reference=w790, "DisabledEnum"=w789) -> ()  [unwired: 1 in, 2 out]
        n404 = property class="Clust (严格)"(reference=w786, "DisabledEnum"=w789) -> ()  [unwired: 1 in, 2 out]
        n405 = Get Date/Time In Seconds() -> (seconds since 1Jan1904=w774:timestamp)
        n406 = Unbundle By Name(w781) -> ("当前滴定数"=w780:sgl)
        n407 = case shown="3" w787 {
          tunnel: w785 -> [w794 w798 w802 w806 w809]
          tunnel: [w793 w797 w801 w805 w810] -> w782
          tunnel: w780 -> [w792 w796 w800 w804 w808]
          tunnel: w774 -> [w791 w795 w799 w803 w807]
          frame 1, Default {
            n408 = Bundle By Name(cluster=w794, "测量吸光度1"=w792, "零点校准时间"=w791) -> (w793:T5)
          }
          frame 2 {
            n409 = Bundle By Name(cluster=w798, "测量吸光度2"=w796, "标液校准时间1"=w795) -> (w797:T5)
          }
          frame 3 {
            n410 = Bundle By Name(cluster=w802, "测量吸光度3"=w800, "标液校准时间2"=w799) -> (w801:T5)
          }
          frame 4 {
            n411 = Bundle By Name(cluster=w806, "测量吸光度4"=w804, "标液校准时间3"=w803) -> (w805:T5)
          }
          frame 5 {
            n412 = Bundle By Name(cluster=w809, "测量吸光度5"=w808, "标液校准时间4"=w807) -> (w810:T5)
          }
        }
        n413 = property class="Clust (严格)"(reference=w784, error in=w783, "Val(Sgnl)"=w782) -> ()  [unwired: 2 out]
        n414 = local read "公式、校准输出"() -> (w778:T6)
        n415 = Bundle By Name(cluster=w778, "校准.校准？"=FALSE ("校准？"), "校准.校准点1-5"=u16 0, "校准.校准浓度"=0.0) -> (w775:T6)
        n416 = global write "CODMn断电保存全局变量.vi" "公式、校准输出"(w775) -> ()
      }
      event "模型选择": Value Change {
        w811 = T10 {"曲线模型"={"标液浓度1"=0.0, "测量吸光度1"=0.0, "样品1启用"=FALSE, "标液浓度2"=0.0, "测量吸光度2"=0.0, "样品2启用"=FALSE, "标液浓度3"=0.0, "测量吸光度3"=0.0, "样品3启用"=FALSE, "标液浓度4"=0.0, "测量吸光度4"=0.0, "样品4启用"=FALSE, "标液浓度5"=0.0, "测量吸光度5"=0.0, "样品5启用"=FALSE, "模型"=enum."线性", "method"=enum."最小二乘", "精度"=7.0, "XY图"=[], "拟合公式"="", "r^2"=0.0, "零点校准时间"=timestamp(0 s since 1904-01-01), "标液校准时间1"=timestamp(0 s since 1904-01-01), "标液校准时间2"=timestamp(0 s since 1904-01-01), "标液校准时间3"=timestamp(0 s since 1904-01-01), "标液校准时间4"=timestamp(0 s since 1904-01-01)}, "Polynomial Coefficients"=[]} ("输出簇")
        n417 = event-data() -> ()  [unwired: 1 in, 6 out]
        n418 = call <vilib>:"Application Directory.vi"() -> ("Application Directory"=w828:path)
        n419 = Build Path(base path=w828, name or relative path="config" ("名称或相对路径")) -> (appended path=w826:path)
        n420 = Concatenate Strings("曲线模型" ("字符串"), ".ini" ("字符串")) -> (w824:string)
        n421 = Build Path(base path=w826, name or relative path=w824) -> (appended path=w829:path)
        n422 = Flatten To String(anything="模型选择") -> (data string=w822:string)  [unwired: 3 in, 2 out]
        n423 = call <vilib>:"Open Config Data.vi"("configuration file path"=w829) -> ("error out"=w832:errorcluster, "refnum"=w833:T12)  [unwired: 8 in, 1 out]
        n424 = call <userlib>:"Read Section Cluster__ogtk.vi"("section (optional)"=w822, "error in (no error)"=w832, "Section Formatted Cluster Type"=w811, "refnum"=w833) -> ("error out"=w830:errorcluster, "Section Formatted Cluster"=w823:variant, "dup refnum"=w831:T12)  [unwired: 3 in, 2 out]
        n425 = call <vilib>:"Close Config Data.vi"("error in (no error)"=w830, "refnum"=w831) -> ()  [unwired: 8 in, 2 out]
        n426 = Variant To Data(type=w811, Variant=w823) -> (data=w820:T10)  [unwired: 1 in, 1 out]
        n427 = Unbundle By Name(w820) -> ("曲线模型"=w812:T5, "Polynomial Coefficients"=w819:dbl[])
        n428 = property class="Clust (严格)"(reference=w813, "Value"=w812) -> ()  [unwired: 1 in, 2 out]
        n429 = Array To Cluster(array=w819) -> (cluster=w818:T15)
        n430 = local read "公式、校准输出"() -> (w815:T6)
        n431 = Bundle By Name(cluster=w815, "公式"=w818, "校准.校准？"=FALSE) -> (w817:T6)
      }
    }
    "公式、校准输出" <- w529
  }
  n432 = while {
    tunnel: w13 -> [_]
    stop <- FALSE stop-if-true
    n433 = global read "VARCODMn全局变量.vi" "状态告警区"() -> (w841:T17)
    n434 = Wait (ms)(milliseconds to wait=u32 500 ("等待时间（毫秒）")) -> ()  [unwired: 1 out]
    n435 = Unbundle By Name(w841) -> ("系统时间"=w834:timestamp, "工作状态"=w840:u16)
    n436 = Bundle By Name(cluster=T23 {"时间源选择"=enum."系统时间源", "外部时间源"=timestamp(0 s since 1904-01-01)} ("时间源"), "时间源选择"=enum16{"系统时间源", "仪器时间源"}."仪器时间源", "外部时间源"=w834) -> (w836:T23)
    n437 = Not Equal?(x=w840, y=T24."空闲") -> (x != y?=w838:bool)
    n438 = property on="定时启动" class="定时设置 (严格)"("仪器状态"=w838, "时间源"=w836) -> ()  [unwired: 2 in, 2 out]
    n439 = vi-ref "斯坦道CODMn新电路板.lvlib:CODMn测量流程.vi"() -> (w847:refnum<vi>)
    n440 = property class="VI"(reference=w847) -> ("Exec.State"=w845:T14, "Name"=w846:string)  [unwired: 1 in, 2 out]
    n441 = Unbundle By Name("定时启动") -> ("启动"=w842:bool, "控制命令"=w843:T8)
    n442 = case shown="真" w842 {
      tunnel: w846 -> [_ w852]
      tunnel: w843 -> [_ w851]
      tunnel: w845 -> [_ w850]
      frame False {
      }
      frame True {
        n443 = case shown="\"Idle\"" w850 {
          tunnel: w852 -> [_ w857]
          tunnel: w851 -> [_ w854]
          frame "Bad", Default {
          }
          frame "Idle" {
            n444 = Increment(x=w854) -> (x+1=w853:T8)
            n445 = Open VI Reference(type specifier VI Refnum (for type only)=refnum<vi> refnum, vi path=w857, options=128 ("选项")) -> (vi reference=w858:refnum<vi>, error out=w859:errorcluster)  [unwired: 3 in]
            n446 = call-by-ref "开始异步调用"(reference=w858, error in=w859, "控制命令"=w853) -> (reference out=w860:refnum<vi>, error out=w861:errorcluster)  [unwired: 11 in]
            n447 = Close Reference(reference=w860, error in (no error)=w861) -> ()  [unwired: 1 out]
          }
        }
      }
    }
  }
  n448 = while {
    shift-right: [w875] -> _
    shift-left: u32 0 ("等待时间（毫秒）") -> [w876]
    stop <- FALSE stop-if-true
    # "密码权限设置"
    n449 = global read "VARCODMn全局变量.vi" "权限等级"() -> (w867:enum16{"一级权限", "二级权限", "三级权限", "超级权限"})
    n450 = property on="公式单个写入" class="Bool"("Visible"=FALSE ("可见")) -> ()  [unwired: 2 in, 2 out]
    n451 = Wait (ms)(milliseconds to wait=u32 1000 ("等待时间（毫秒）")) -> ()  [unwired: 1 out]
    n452 = case shown="真" "布尔" {
      tunnel: w876 -> [_ w900]
      tunnel: [_ w899] -> w875
      frame False {
      }
      frame True {
        n453 = Increment(x=w900) -> (x+1=w899:u32)
      }
    }
    n454 = case shown="\"一级权限\", 默认" w867 {
      tunnel: [T22."Disabled and Grayed Out" ("f") T22."Enabled" ("禁用") w894 w897] -> w870
      tunnel: [T22."Disabled and Grayed Out" ("f") T22."Disabled and Grayed Out" ("f") w894 w897] -> w871
      tunnel: [FALSE ("可见") TRUE ("可见") TRUE ("可见") TRUE ("可见")] -> w866
      tunnel: ["一级权限" "二级权限" "三级权限" "超级权限"] -> w865
      tunnel: [TRUE _ _ _] -> w864
      frame "一级权限", Default {
      }
      frame "二级权限" {
      }
      frame "三级权限" {
        w894 = T22."Enabled" ("禁用")
      }
      frame "超级权限" {
        w897 = T22."Enabled" ("禁用")
      }
    }
    "权限等级" <- w865
    n455 = local read "量程下拉列表"() -> (w869:enum16{"低量程1", "低量程2", "高量程1", "高量程2"})
    n456 = case shown="\"高量程2\"" w869 {
      tunnel: [TRUE ("可见") FALSE ("可见") TRUE ("可见") FALSE ("可见")] -> w868
      frame "低量程1", Default {
      }
      frame "低量程2" {
      }
      frame "高量程1" {
      }
      frame "高量程2" {
      }
    }
    n457 = Greater Or Equal?(x=w875, y=u32 3600) -> (x >= y?=w873:bool)
    n458 = case shown="真" w873 {
      frame False {
      }
      frame True {
        n459 = global write "VARCODMn全局变量.vi" "权限等级"(enum16{"一级权限", "二级权限", "三级权限", "超级权限"}."一级权限" ("权限等级")) -> ()
      }
    }
    n460 = property on="公式切换阈值滴定数(0~9999)" class="DigNum (严格)"("Visible"=w868) -> ()  [unwired: 2 in, 2 out]
    n461 = Not(x=w864) -> (.not. x?=w862:bool)
    n462 = property on="写公式" class="Bool"("DisabledEnum"=w870) -> ()  [unwired: 2 in, 2 out]
    n463 = property on="流程固件" class="Bool"("DisabledEnum"=w871) -> ()  [unwired: 2 in, 2 out]
    n464 = property on="平台反控标样校准" class="Enum (严格)"("Visible"=w866) -> ()  [unwired: 2 in, 2 out]
    n465 = property on="平台反控校准量程" class="Enum (严格)"("Visible"=w866) -> ()  [unwired: 2 in, 2 out]
    n466 = property on="布尔" class="Bool (严格)"("Value"=w862) -> ()  [unwired: 2 in, 2 out]
    n467 = property on="关键参数设置" class="Bool"("Visible"=w866) -> ()  [unwired: 2 in, 2 out]
    n468 = property on="量程参数设置" class="Bool"("Visible"=w866) -> ()  [unwired: 2 in, 2 out]
    n469 = property on="试剂余量设置" class="Bool"("Visible"=w866) -> ()  [unwired: 2 in, 2 out]
    n470 = property on="串口设置" class="Bool"("Visible"=w866) -> ()  [unwired: 2 in, 2 out]
    n471 = property on="模块启用" class="Bool (严格)"("Visible"=w866) -> ()  [unwired: 2 in, 2 out]
    n472 = property on="流程固件" class="Bool"("Visible"=w866) -> ()  [unwired: 2 in, 2 out]
  }
  n473 = while {
    tunnel: w44 -> [w908]
    tunnel: w55 -> [_]
    stop <- FALSE stop-if-true
    n474 = global read "CODMn断电保存全局变量.vi" "流程路径"() -> (w907:path)
    n475 = Get Queue Status(queue=w908) -> (queue out=w904:refnum<queue>, # elements in queue=w903:i32)  [unwired: 2 in, 6 out]
    n476 = local write "流程路径"(w907) -> ()
    n477 = case shown="0" w903 {
      tunnel: w904 -> [_ w927]
      frame Default {
      }
      frame 0 {
        w915 = u16 0 items=["空闲"=0, "水样测试"=1, "标样核查"=2, "零点核查"=3, "跨度核查"=4, "空白测试"=5, "平行样测试"=6, "加标回收"=7, "空白校准"=8, "标样校准"=9, "初始化（清洗）"=10, "调试"=22, "填充管路"=30, "清洗管路"=31, "清洗反应杯"=32] ("工作状态")
        # "试剂填充 172 \n管路清洗108\n氨氮92\n总磷131\n总磷海水147\n总氮76\n总氮海水92"
        n478 = global read "VARCODMn全局变量.vi" "状态告警区"() -> (w917:T17)
        n479 = global read "CODMn断电保存全局变量.vi" "站号"() -> (w916:u16)
        n480 = Unbundle By Name(w917) -> ("系统时间"=w923:timestamp, "工作状态"=w914:u16)
        n481 = Bundle By Name(cluster=cluster{"命令":string, "data":variant} {"命令"="", "data"=variant} ("元素"), "命令"="读状态告警区", "data"=w916) -> (w925:cluster{"命令":string, "data":variant})
        n482 = Get Date/Time In Seconds() -> (seconds since 1Jan1904=w922:timestamp)
        n483 = Subtract(x=w922, y=w923) -> (x-y=w921:dbl)
        n484 = Equal?(x=w914, y=w915) -> (x = y?=w913:bool)
        n485 = Enqueue Element(queue=w927, element=w925) -> (queue out=w912:refnum<queue>)  [unwired: 2 in, 2 out]
        n486 = case shown="真" w913 {
          tunnel: w916 -> [_ w932]
          tunnel: w912 -> [w928 w930]
          tunnel: [w928 w929] -> w911
          frame False {
          }
          frame True {
            n487 = Bundle By Name(cluster=cluster{"命令":string, "data":variant} {"命令"="", "data"=variant} ("元素"), "命令"="读测量数据区", "data"=w932) -> (w931:cluster{"命令":string, "data":variant})
            n488 = Enqueue Element(queue=w930, element=w931) -> (queue out=w929:refnum<queue>)  [unwired: 2 in, 2 out]
          }
        }
        n489 = Absolute Value(x=w921) -> (abs(x)=w920:dbl)
        n490 = Greater Or Equal?(x=w920, y=120.0) -> (x >= y?=w918:bool)
        n491 = case shown="真" w918 {
          tunnel: w911 -> [_ w939]
          tunnel: w916 -> [_ w937]
          frame False {
          }
          frame True {
            n492 = Bundle By Name(cluster=T25 {"站号"=21, "量程切换"=enum."AUTO", "控制命令"=13, "模式设置"=enum."待机", "测量间隔"=0} ("参数"), "站号"=w937) -> (w935:T25)
            n493 = call "CODMn启动命令.vi"("参数"=w935) -> ("启动命令"=w938:cluster{"命令":string, "data":variant})  [unwired: 10 in]
            n494 = Enqueue Element(queue=w939, element=w938) -> ()  [unwired: 2 in, 3 out]
          }
        }
      }
    }
    n495 = global read "CODMn断电保存全局变量.vi" "MB通信方式选择"() -> (w905:enum16{"串口", "TCP"})
    n496 = case shown="\"TCP\"" w905 {
      tunnel: [w940 w941] -> w906
      frame "串口", Default {
        n497 = global read "CODMn断电保存全局变量.vi" "VISA Resource"() -> (w940:refnum<visa-resource-name>)
      }
      frame "TCP" {
        n498 = global read "CODMn断电保存全局变量.vi" "IP"() -> (w941:string)
      }
    }
    "字符串" <- w906
    n499 = Wait (ms)(milliseconds to wait=u32 1000 ("等待时间（毫秒）")) -> ()  [unwired: 1 out]
    n500 = global read "CODMn断电保存全局变量.vi" "远程校准量程"() -> (w901:enum16{"低量程1", "低量程2", "高量程1", "高量程2"})
    n501 = global read "CODMn断电保存全局变量.vi" "远程标样校准"() -> (w902:enum16{"标液1", "标液2", "标液3", "标液4"})
    n502 = local write "平台反控校准量程"(w901) -> ()
    n503 = local write "平台反控标样校准"(w902) -> ()
  }
  n504 = call "校准中 (子VI).vi"("校准按钮"=w43, "曲线模型"=w42) -> ()  [unwired: 10 in]
  n505 = while {
    tunnel: w44 -> [w950]
    tunnel: w54 -> [w949]
    tunnel: w53 -> [w948]
    tunnel: w52 -> [w947]
    tunnel: w51 -> [w946]
    tunnel: w46 -> [w945]
    tunnel: [w944] -> _
    tunnel: w3 -> [w943]
    tunnel: w2 -> [w942]
    stop <- FALSE stop-if-true
    n506 = event shown="[3] \"流程固件\": 值改变" {
      selector: _ -> [_ _ _ _ _ _ _ _ _ _ _ _ _ _ _ _ _ _ _ _ _ _ _ _ _ _ _]
      dyn-events: _ -> [_ _ _ _ _ _ _ _ _ _ _ _ _ _ _ _ _ _ _ _ _ _ _ _ _ _ _]
      timeout: _ -> [_ _ _ _ _ _ _ _ _ _ _ _ _ _ _ _ _ _ _ _ _ _ _ _ _ _ _]
      tunnel: w950 -> [_ _ _ _ _ w983 _ w999 _ _ _ _ _ _ w1080 _ w1104 _ _ _ _ _ _ _ _ _ _]
      tunnel: w949 -> [_ _ _ _ w964 _ _ _ _ w1014 _ _ _ _ _ _ _ _ _ _ _ _ _ _ _ _ _]
      tunnel: w948 -> [_ _ _ _ w963 _ _ _ _ w1010 _ _ _ _ _ _ _ _ _ _ _ _ _ _ _ w1178 w1184]
      tunnel: w947 -> [_ _ _ _ w962 _ _ _ _ w1012 _ _ _ _ _ _ _ _ _ _ _ _ _ _ _ _ _]
      tunnel: w946 -> [_ _ _ _ w965 _ _ _ _ w1008 _ _ _ _ _ _ _ _ _ _ _ _ _ _ _ _ _]
      tunnel: w945 -> [_ _ _ _ _ _ _ _ _ _ _ _ _ _ _ _ w1107 _ _ _ _ _ _ _ _ _ _]
      tunnel: [_ _ _ _ w960 _ _ _ _ _ _ _ _ _ _ _ _ _ _ _ _ _ _ _ _ _ _] -> w944
      tunnel: w943 -> [_ _ _ _ _ _ _ _ _ _ _ _ _ _ _ _ _ w1109 _ _ _ _ _ _ _ _ _]
      tunnel: w942 -> [_ _ _ _ _ _ _ _ _ _ _ _ _ _ _ _ _ _ w1112 _ _ _ _ _ _ _ _]
      event Timeout {
        n507 = event-data() -> ()  [unwired: 1 in, 3 out]
      }
      event "布尔": Value Change {
        n508 = event-data() -> ("NewVal"=w952:bool)  [unwired: 1 in, 5 out]
        n509 = case shown="假" w952 {
          frame False {
            n510 = global write "VARCODMn全局变量.vi" "权限等级"(enum16{"一级权限", "二级权限", "三级权限", "超级权限"}."一级权限" ("权限等级")) -> ()
          }
          frame True {
            n511 = global read "VARCODMn全局变量.vi" "权限密码"() -> (w956:u32[])
            n512 = global read "VARCODMn全局变量.vi" "权限等级"() -> (w955:enum16{"一级权限", "二级权限", "三级权限", "超级权限"})
            n513 = call "密码权限设置.vi"("权限输入"=w955, "权限密码"=w956) -> ("权限输出"=w954:enum16{"一级权限", "二级权限", "三级权限", "超级权限"})  [unwired: 9 in]
            n514 = global write "VARCODMn全局变量.vi" "权限等级"(w954) -> ()
          }
        }
      }
      event "权限等级": Mouse Down {
        n515 = event-data() -> ()  [unwired: 1 in, 8 out]
        n516 = global read "VARCODMn全局变量.vi" "权限密码"() -> (w959:u32[])
        n517 = global read "VARCODMn全局变量.vi" "权限等级"() -> (w958:enum16{"一级权限", "二级权限", "三级权限", "超级权限"})
        n518 = call "密码权限设置.vi"("权限输入"=w958, "权限密码"=w959) -> ("权限输出"=w957:enum16{"一级权限", "二级权限", "三级权限", "超级权限"})  [unwired: 9 in]
        n519 = global write "VARCODMn全局变量.vi" "权限等级"(w957) -> ()
      }
      event "流程固件": Value Change {
        n520 = event-data() -> ()  [unwired: 1 in, 6 out]
        n521 = call "流程固件设置对话框.vi"() -> ()  [unwired: 12 in]
      }
      event "测量模式下拉列表", "量程下拉列表", "参数下拉列表": Value Change {
        n522 = event-data() -> ()  [unwired: 1 in, 6 out]
        n523 = property class="Enum (严格)"(reference=w962) -> ("Value"=w966:T7)  [unwired: 1 in, 2 out]
        n524 = property class="Enum (严格)"(reference=w963) -> ("Value"=w969:enum16{"CODMn"})  [unwired: 1 in, 2 out]
        n525 = property class="Enum (严格)"(reference=w964) -> ("Value"=w968:enum16{"低量程1", "低量程2", "高量程1", "高量程2"})  [unwired: 1 in, 2 out]
        n526 = call "公式读取.vi"("量程"=w968, "测量模式"=w966, "测量参数"=w969) -> ("error out"=w960:errorcluster, "临界滴定数"=w961:dbl, "公式"=w967:cluster{"X^2":dbl, "X":dbl, "b":dbl})  [unwired: 6 in]
        n527 = property class="Clust (严格)"(reference=w965, "Value"=w967) -> ()  [unwired: 1 in, 2 out]
        n528 = local write "公式切换阈值滴定数(0~9999)"(w961) -> ()
        n529 = local read "测量模式下拉列表"() -> (w972:T7)
        n530 = local read "参数下拉列表"() -> (w971:enum16{"CODMn"})
        n531 = local read "量程下拉列表"() -> (w973:enum16{"低量程1", "低量程2", "高量程1", "高量程2"})
        n532 = Bundle("参数下拉列表"=w971, "测量模式下拉列表"=w972, "量程下拉列表"=w973) -> (w970:T26)  [unwired: 1 in]
        n533 = property on="模型选择" class="Clust (严格)"("Val(Sgnl)"=w970) -> ()  [unwired: 2 in, 2 out]
      }
      event "串口设置": Value Change {
        n534 = event-data() -> ()  [unwired: 1 in, 6 out]
        n535 = global read "CODMn断电保存全局变量.vi" "MB通信方式选择"() -> (w974:enum16{"串口", "TCP"})
        n536 = global read "CODMn断电保存全局变量.vi" "VISA Resource"() -> (w980:refnum<visa-resource-name>)
        n537 = global read "CODMn断电保存全局变量.vi" "PORT"() -> (w978:string)
        n538 = global read "CODMn断电保存全局变量.vi" "IP"() -> (w979:string)
        n539 = call "串口配置.vi"("PORT"=w978, "IP"=w979, "MB通信方式选择"=w974, "请选择串口:"=w980) -> ("PORT 2"=w976:string, "IP 2"=w977:string, "确认 2"=w981:bool, "VISA资源名称 2"=w982:refnum<visa-resource-name>, "MB通信方式选择 2"=w975:enum16{"串口", "TCP"})  [unwired: 3 in]
        n540 = case shown="真" w981 {
          tunnel: w982 -> [_ w988]
          tunnel: w983 -> [_ w987]
          tunnel: w977 -> [_ w986]
          tunnel: w976 -> [_ w985]
          tunnel: w975 -> [_ w984]
          frame False {
          }
          frame True {
            n541 = flat-sequence {
              tunnel: w988 -> [w993]
              tunnel: w987 -> [w994]
              tunnel: w986 -> [w992]
              tunnel: w985 -> [w991]
              tunnel: w984 -> [w990]
              frame #0 {
                n542 = global write "CODMn断电保存全局变量.vi" "IP"(w992) -> ()
                n543 = global write "CODMn断电保存全局变量.vi" "PORT"(w991) -> ()
                n544 = global write "CODMn断电保存全局变量.vi" "VISA Resource"(w993) -> ()
                n545 = global write "CODMn断电保存全局变量.vi" "MB通信方式选择"(w990) -> ()
                n546 = Flush Queue(queue=w994) -> (queue out=w989:refnum<queue>)  [unwired: 1 in, 2 out]
                n547 = Enqueue Element(queue=w989, element=cluster{"命令":string, "data":variant} {"命令"="启用模块", "data"=variant} ("元素")) -> ()  [unwired: 2 in, 3 out]
              }
              frame #1 {
                n548 = call "配置文件保存.vi"() -> ()  [unwired: 12 in]
              }
            }
          }
        }
      }
      event "平台反控校准量程", "平台反控标样校准": Value Change {
        n549 = event-data() -> ()  [unwired: 1 in, 6 out]
        n550 = flat-sequence {
          frame #0 {
            n551 = global write "CODMn断电保存全局变量.vi" "远程校准量程"("平台反控校准量程") -> ()
            n552 = global write "CODMn断电保存全局变量.vi" "远程标样校准"("平台反控标样校准") -> ()
          }
          frame #1 {
            n553 = call "配置文件保存.vi"() -> ()  [unwired: 12 in]
          }
        }
      }
      event "模块启用": Value Change {
        n554 = event-data() -> ("OldVal"=w1000:bool)  [unwired: 1 in, 5 out]
        n555 = Flush Queue(queue=w999) -> (queue out=w998:refnum<queue>)  [unwired: 1 in, 2 out]
        n556 = case shown="假" w1000 {
          tunnel: w998 -> [w1001 w1003]
          frame False {
            n557 = Enqueue Element(queue=w1001, element=cluster{"命令":string, "data":variant} {"命令"="停用模块", "data"=variant} ("元素")) -> ()  [unwired: 2 in, 3 out]
          }
          frame True {
            n558 = Enqueue Element(queue=w1003, element=cluster{"命令":string, "data":variant} {"命令"="启用模块", "data"=variant} ("元素")) -> ()  [unwired: 2 in, 3 out]
          }
        }
      }
      event "流程路径": Value Change {
        n559 = event-data() -> ()  [unwired: 1 in, 6 out]
        n560 = flat-sequence {
          frame #0 {
            n561 = local read "流程路径"() -> (w1005:path)
            n562 = global write "CODMn断电保存全局变量.vi" "流程路径"(w1005) -> ()
          }
          frame #1 {
            n563 = call "配置文件保存.vi"() -> ()  [unwired: 12 in]
          }
        }
      }
      event "公式单个写入": Value Change {
        n564 = event-data() -> ()  [unwired: 1 in, 6 out]
        n565 = property class="Enum (严格)"(reference=w1014) -> ("Value"=w1013:enum16{"低量程1", "低量程2", "高量程1", "高量程2"})  [unwired: 1 in, 2 out]
        n566 = property class="Enum (严格)"(reference=w1012) -> ("Value"=w1011:T7)  [unwired: 1 in, 2 out]
        n567 = property class="Enum (严格)"(reference=w1010) -> ("Value"=w1009:enum16{"CODMn"})  [unwired: 1 in, 2 out]
        n568 = property class="Clust (严格)"(reference=w1008) -> ("Value"=w1007:cluster{"X^2":dbl, "X":dbl, "b":dbl})  [unwired: 1 in, 2 out]
        n569 = call "公式写入.vi"("公式"=w1007, "量程"=w1013, "测量模式"=w1011, "测量参数"=w1009) -> ("error out"=w1015:errorcluster)  [unwired: 7 in]
        n570 = case shown="无错误" w1015 {
          tunnel: w1011 -> [w1024 _]
          tunnel: w1013 -> [w1022 _]
          tunnel: w1007 -> [w1018 _]
          tunnel: ["写入成功" ("消息") "写入失败" ("消息")] -> w1006
          frame No Error {
            n571 = Equal?(x=w1022, y=enum16{"低量程", "高量程"}."低量程" ("量程下拉列表")) -> (x = y?=w1020:bool)
            n572 = Equal?(x=w1024, y=T7."水样测量") -> (x = y?=w1021:bool)
            n573 = And(x=w1021, y=w1020) -> (x .and. y?=w1019:bool)
            n574 = case shown="真" w1019 {
              tunnel: w1018 -> [_ w1025]
              frame False {
              }
              frame True {
                n575 = Unbundle By Name(w1025) -> ("X^2"=w1028:dbl, "X"=w1027:dbl, "b"=w1026:dbl)
                n576 = global read "CODMn断电保存全局变量.vi" "CODMn仪器参数"() -> (w1029:T27)
                n577 = Bundle By Name(cluster=w1029, "曲线截距"=w1026, "曲线斜率"=w1027, "二次多项式系数"=w1028) -> (w1030:T27)
                n578 = global write "CODMn断电保存全局变量.vi" "CODMn仪器参数"(w1030) -> ()
              }
            }
          }
          frame Error {
          }
        }
        n579 = One Button Dialog(message=w1006) -> ()  [unwired: 1 in, 1 out]
      }
      event "公式、校准输出": Value Change {
        n580 = event-data() -> ()  [unwired: 1 in, 6 out]
        n581 = local read "公式、校准输出"() -> (w1033:T6)
        n582 = Unbundle By Name(w1033) -> ("公式"=w1032:cluster{"X^2":dbl, "X":dbl, "B":dbl})
        n583 = local write "公式"(w1032) -> ()
      }
      event "量程参数设置": Value Change {
        n584 = event-data() -> ()  [unwired: 1 in, 6 out]
        n585 = global read "VARCODMn全局变量.vi" "MB session in"() -> (w1036:refnum<class "MB_Master.lvclass">)
        n586 = call "读取量程参数.vi"("引用选择"=enum16{"MB引用", "自建引用"}."MB引用", "MB session in"=w1036) -> ("自动测试量程配置"=w1034:T29)  [unwired: 7 in, 2 out]
        n587 = global read "CODMn断电保存全局变量.vi" "质控参数设置"() -> (w1037:T30)
        n588 = call "量程参数设置.vi"("自动测试量程配置"=w1034, "质控参数设置"=w1037) -> ("checkout"=w1040:bool, "自动测试量程配置 2"=w1039:T31, "输出簇"=w1038:T32)  [unwired: 7 in]
        n589 = case shown="真" w1040 {
          tunnel: w1039 -> [_ w1044]
          tunnel: w1038 -> [_ w1043]
          tunnel: w1037 -> [_ w1042]
          frame False {
          }
          frame True {
            n590 = flat-sequence {
              tunnel: w1044 -> [w1046]
              tunnel: w1043 -> [w1049]
              tunnel: w1042 -> [w1048]
              tunnel: [w1045] -> w1041
              tunnel: w1041 -> [_]
              frame #0 {
                n591 = global write "CODMn断电保存全局变量.vi" "自动测试量程配置"(w1046) -> ()
                n592 = Unbundle By Name(w1049) -> ("跨度值"=w1054:dbl, "零点标准液浓度"=w1053:dbl, "跨度标准液浓度"=w1052:dbl, "标准液标准浓度"=w1051:dbl)
                n593 = Bundle By Name(cluster=w1048, "跨度值"=w1054, "零点标准液浓度"=w1053, "跨度标准液浓度"=w1052, "标准液标准浓度"=w1051) -> (w1050:T30)
                n594 = global read "VARCODMn全局变量.vi" "MB session in"() -> (w1047:refnum<class "MB_Master.lvclass">)
                n595 = global write "CODMn断电保存全局变量.vi" "质控参数设置"(w1050) -> ()
                n596 = call "写入量程参数.vi"("自动测试量程配置"=w1046, "MB session in"=w1047) -> ("error out"=w1045:errorcluster)  [unwired: 8 in, 1 out]
              }
              frame #1 {
                n597 = call "配置文件保存.vi"() -> ()  [unwired: 12 in]
              }
            }
          }
        }
      }
      event "关键参数设置": Value Change {
        n598 = event-data() -> ()  [unwired: 1 in, 6 out]
        n599 = global read "CODMn断电保存全局变量.vi" "CODMn仪器参数"() -> (w1055:T27)
        n600 = call "仪器参数设置.vi"("氨氮仪器参数"=w1055) -> ("仪器参数设置输出"=w1056:T33)  [unwired: 10 in]
        n601 = Unbundle By Name(w1056) -> ("确定"=w1057:bool)
        n602 = case shown="真" w1057 {
          tunnel: w1056 -> [_ w1059]
          tunnel: w1055 -> [_ w1058]
          frame False {
          }
          frame True {
            n603 = flat-sequence {
              tunnel: w1059 -> [w1076]
              tunnel: w1058 -> [w1075]
              frame #0 {
                n604 = Unbundle By Name(w1076) -> ("测量量程"=w1074:dbl, "测量精度"=w1073:dbl, "测量间隔"=w1072:dbl, "消解温度"=w1071:dbl, "消解时长"=w1069:dbl, "空白校准时间"=w1068:timestamp, "曲线截距"=w1067:dbl, "曲线斜率"=w1066:dbl, "测量检出限"=w1065:dbl, "测量信号值"=w1064:dbl, "线性相关系数"=w1063:dbl, "二次多项式系数"=w1062:dbl, "标样校准时间"=w1061:timestamp, "稀释倍数"=w1060:dbl)
                n605 = Bundle By Name(cluster=w1075, "测量量程"=w1074, "测量精度"=w1073, "测量间隔"=w1072, "消解温度"=w1071, "消解时长"=w1069, "空白校准时间"=w1068, "曲线截距"=w1067, "曲线斜率"=w1066, "测量检出限"=w1065, "测量信号值"=w1064, "线性相关系数"=w1063, "二次多项式系数"=w1062, "标样校准时间"=w1061, "稀释倍数"=w1060) -> (w1070:T27)
                n606 = global write "CODMn断电保存全局变量.vi" "CODMn仪器参数"(w1070) -> ()
              }
              frame #1 {
                n607 = call "配置文件保存.vi"() -> ()  [unwired: 12 in]
              }
            }
          }
        }
      }
      event "试剂余量设置": Value Change {
        n608 = event-data() -> ()  [unwired: 1 in, 6 out]
        n609 = call "试剂余量显示UI.vi"() -> ()  [unwired: 12 in]
      }
      event "手动启动": Value Change {
        n610 = event-data() -> ()  [unwired: 1 in, 6 out]
        n611 = call "CODMn启动参数对话框.vi"() -> ("标样浓度输出"=w1078:dbl, "确认"=w1077:bool, "元素"=w1079:cluster{"命令":string, "data":variant})  [unwired: 9 in]
        n612 = case shown="真" w1077 {
          tunnel: w1080 -> [_ w1090]
          tunnel: w1079 -> [_ w1089]
          tunnel: w1078 -> [_ w1082]
          frame False {
          }
          frame True {
            (unwired) u16 31 ("y")
            n613 = Enqueue Element(queue=w1090, element=w1089) -> ()  [unwired: 2 in, 3 out]
            n614 = Unbundle By Name(w1089) -> ("data"=w1088:variant)
            n615 = global write "VARCODMn全局变量.vi" "手动启动"(TRUE ("手动启动")) -> ()
            n616 = Variant To Data(type=cluster{"站号":u16, "控制命令":u16[]} {"站号"=0, "控制命令"=[]} ("输出簇"), Variant=w1088) -> (data=w1086:cluster{"站号":u16, "控制命令":u16[]})  [unwired: 1 in, 1 out]
            n617 = Unbundle By Name(w1086) -> ("控制命令"=w1085:u16[])
            n618 = Index Array(array=w1085) -> (element=w1084:u16)  [unwired: 1 in]
            n619 = Swap Bytes(anything=w1084) -> (byte swapped=w1083:u16)
            n620 = case shown="9" w1083 {
              tunnel: w1082 -> [_ w1091 _ _ _]
              frame 0, Default {
              }
              frame 2 {
                # "标样核查"
                n621 = flat-sequence {
                  tunnel: w1091 -> [w1092]
                  frame #0 {
                    n622 = global read "CODMn断电保存全局变量.vi" "质控参数设置"() -> (w1094:T30)
                    n623 = Bundle By Name(cluster=w1094, "标准液标准浓度"=w1092) -> (w1093:T30)
                    n624 = global write "CODMn断电保存全局变量.vi" "质控参数设置"(w1093) -> ()
                  }
                  frame #1 {
                    n625 = call "配置文件保存.vi"() -> ()  [unwired: 12 in]
                  }
                }
              }
              frame 8 {
                # "空白校准"
                n626 = property on="校准1" class="Bool (严格)"("Val(Sgnl)"=TRUE ("值(信号)")) -> ()  [unwired: 2 in, 2 out]
                n627 = property on="量程下拉列表" class="Enum (严格)"("Val(Sgnl)"=enum16{"低量程1", "低量程2", "高量程1", "高量程2"}."低量程1" ("值(信号)")) -> ()  [unwired: 2 in, 2 out]
              }
              frame 9 {
                # "标样校准"
                n628 = local read "平台反控标样校准"() -> (w1099:enum16{"标液1", "标液2", "标液3"})
                n629 = case shown="\"标液3\"" w1099 {
                  tunnel: TRUE -> [w1100 w1101 w1102]
                  frame "标液1", Default {
                    n630 = property on="校准2" class="Bool (严格)"("Val(Sgnl)"=w1100) -> ()  [unwired: 2 in, 2 out]
                  }
                  frame "标液2" {
                    n631 = property on="校准3" class="Bool (严格)"("Val(Sgnl)"=w1101) -> ()  [unwired: 2 in, 2 out]
                  }
                  frame "标液3" {
                    n632 = property on="校准4" class="Bool (严格)"("Val(Sgnl)"=w1102) -> ()  [unwired: 2 in, 2 out]
                  }
                }
                n633 = local read "平台反控校准量程"() -> (w1097:enum16{"低量程1", "低量程2", "高量程1", "高量程2"})
                n634 = property on="量程下拉列表" class="Enum (严格)"("Val(Sgnl)"=w1097) -> ()  [unwired: 2 in, 2 out]
              }
              frame 31 {
                n635 = One Button Dialog(message="“请将试剂管,水样管,标样管等管路置于纯水中”" ("消息")) -> ()  [unwired: 1 in, 1 out]
              }
            }
          }
        }
      }
      event "单步测试": Value Change {
        n636 = event-data() -> ()  [unwired: 1 in, 6 out]
        n637 = call "COMn单步调试对话框.vi"() -> ()  [unwired: 12 in]
      }
      event "停止": Value Change {
        n638 = event-data() -> ()  [unwired: 1 in, 6 out]
        n639 = Cancel Notification(0:w1107) -> (8:w1108:refnum<notifier>)  [unwired: 1 in, 2 out]
        n640 = Send Notification(notification=TRUE ("通知"), notifier=w1108) -> ()  [unwired: 1 in, 2 out]
        n641 = Enqueue Element(queue=w1104, element=cluster{"命令":string, "data":variant} {"命令"="启动", "data"=variant(cluster{"站号":u16, "控制命令":u16[]} {"站号"=21, "控制命令"=[2816]})} ("启动命令")) -> ()  [unwired: 2 in, 3 out]
      }
      event "设置", "参数查询": Value Change {
        n642 = event-data() -> ()  [unwired: 1 in, 6 out]
        n643 = property on="窗格" class="Pane"("Origin"=T13 {"Horizontal"=0, "Vertical"=628} ("原点")) -> ()  [unwired: 2 in, 2 out]
        n644 = invoke on="子面板" class="SubPnl" method="Remove VI"() -> (error out=w1110:errorcluster)  [unwired: 3 in, 2 out]
        n645 = invoke on="子面板" class="SubPnl" method="Insert VI"(error in=w1110, "VI Ref"=w1109) -> ()  [unwired: 2 in, 4 out]
      }
      event "仪器校准": Value Change {
        n646 = event-data() -> ()  [unwired: 1 in, 6 out]
        n647 = invoke on="子面板" class="SubPnl" method="Remove VI"() -> (error out=w1113:errorcluster)  [unwired: 3 in, 2 out]
        n648 = invoke on="子面板" class="SubPnl" method="Insert VI"(error in=w1113, "VI Ref"=w1112) -> ()  [unwired: 2 in, 4 out]
      }
      event "滴定曲线": Value Change {
        n649 = event-data() -> ()  [unwired: 1 in, 6 out]
        n650 = vi-ref "读取CODMn数据波形新.vi"() -> (w1115:refnum<vi>)
        n651 = property class="VI"(reference=w1115) -> ("Name"=w1121:string)  [unwired: 1 in, 2 out]
        n652 = Open VI Reference(type specifier VI Refnum (for type only)=refnum<vi> refnum, vi path=w1121, options=128 ("选项")) -> (vi reference=w1119:refnum<vi>, error out=w1118:errorcluster)  [unwired: 3 in]
        n653 = call-by-ref "?"(reference=w1119, error in=w1118) -> (reference out=w1116:refnum<vi>, error out=w1117:errorcluster)  [unwired: 12 in]
        n654 = Close Reference(reference=w1116, error in (no error)=w1117) -> ()  [unwired: 1 out]
      }
      event "历史波形", "历史波形 2": Value Change {
        n655 = event-data() -> ("CtlRef"=w1123:refnum<vi>)  [unwired: 1 in, 5 out]
        n656 = property class="Bool (严格)"(reference=w1123) -> ("Label.Text"=w1122:string)  [unwired: 1 in, 2 out]
        n657 = call-poly <vilib>:"Read Waveforms from File.vi"() -> ("error out"=w1124:errorcluster, "first waveform in record"=w1125:waveform(dbl))  [unwired: 6 in, 2 out]
        n658 = case shown="无错误" w1124 {
          tunnel: w1125 -> [w1129 _]
          tunnel: w1122 -> [w1126 _]
          frame No Error {
            n659 = Unbundle By Name(w1129) -> ("t0"=w1128:timestamp, "Y"=w1127:dbl[])  [unwired: 2 out]
            n660 = case shown="\"历史波形2\"" w1126 {
              tunnel: w1128 -> [w1130 w1133]
              tunnel: w1127 -> [w1131 w1132]
              frame "历史波形2" {
                n661 = global write "VARCODMn全局变量.vi" "温度波形时间"(w1130) -> ()
                n662 = global write "VARCODMn全局变量.vi" "时间-温度"(w1131) -> ()
                n663 = global write "VARCODMn全局变量.vi" "温度曲线"(w1131) -> ()
              }
              frame "历史波形", Default {
                n664 = global write "VARCODMn全局变量.vi" "波形时间"(w1133) -> ()
                n665 = global write "VARCODMn全局变量.vi" "ORP滴定曲线"(w1132) -> ()
                n666 = global write "VARCODMn全局变量.vi" "滴定数-ORP值"(w1132) -> ()
              }
            }
          }
          frame Error {
            n667 = One Button Dialog(message="打开失败" ("消息")) -> ()  [unwired: 1 in, 1 out]
          }
        }
      }
      event "返回", "返回 2", "返回 3": Value Change {
        n668 = event-data() -> ()  [unwired: 1 in, 6 out]
        n669 = property on="窗格" class="Pane"("Origin"=T13 {"Horizontal"=0, "Vertical"=0} ("原点")) -> ()  [unwired: 2 in, 2 out]
      }
      event "公式.X^2", "公式.X", "公式.b", "公式切换阈值滴定数(0~9999)": Mouse Down {
        n670 = event-data() -> ("CtlRef"=w1139:refnum<vi>)  [unwired: 1 in, 5 out]
        n671 = property class="DigNum (严格)"(reference=w1139) -> (reference out=w1137:refnum<vi>, "Value"=w1138:dbl)  [unwired: 1 in, 1 out]
        n672 = call "数字键盘.vi"("OldNumber"=w1138) -> ("NewNumber"=w1136:dbl)
        n673 = property class="DigNum (严格)"(reference=w1137, "Val(Sgnl)"=w1136) -> ()  [unwired: 1 in, 2 out]
      }
      event "读公式": Value Change {
        n674 = event-data() -> ()  [unwired: 1 in, 6 out]
      }
      event "写公式": Value Change {
        n675 = event-data() -> ()  [unwired: 1 in, 6 out]
        n676 = Two Button Dialog(message="即将将左侧拟合公式写入仪器所有模式\n请选择是否写入?" ("消息"), 1:"否" ("F按钮名称（“取消”）"), 2:"是" ("T按钮名称（“确定”）")) -> (T button?=w1140:bool)
        n677 = case shown="真" w1140 {
          frame False {
          }
          frame True {
            n678 = for {
              N: 7 -> [_]
              shift-right: [w1153] -> _
              shift-left: T7."水样测量" ("测量模式下拉列表") -> [w1154]
              tunnel: [w1152] -> w1148
              n679 = call "公式写入.vi"("临界滴定数"="公式切换阈值滴定数(0~9999)", "公式"="公式", "量程"="量程下拉列表", "测量模式"=w1154, "测量参数"="参数下拉列表") -> ("error out"=w1158:errorcluster)  [unwired: 6 in]
              n680 = Increment(x=w1154) -> (x+1=w1153:T7)
              n681 = case shown="无错误" w1158 {
                tunnel: w1154 -> [w1167 _]
                tunnel: "量程下拉列表" -> [w1166 _]
                tunnel: "公式" -> [w1162 _]
                tunnel: ["写入成功" ("消息") "写入失败" ("消息")] -> w1152
                frame No Error {
                  n682 = Equal?(x=w1166, y=enum16{"低量程1", "低量程2", "高量程1", "高量程2"}."低量程1") -> (x = y?=w1164:bool)
                  n683 = Equal?(x=w1167, y=T7."水样测量") -> (x = y?=w1165:bool)
                  n684 = And(x=w1165, y=w1164) -> (x .and. y?=w1163:bool)
                  n685 = case shown="真" w1163 {
                    tunnel: w1162 -> [_ w1168]
                    frame False {
                    }
                    frame True {
                      n686 = Unbundle By Name(w1168) -> ("X^2"=w1171:dbl, "X"=w1170:dbl, "b"=w1169:dbl)
                      n687 = global read "CODMn断电保存全局变量.vi" "CODMn仪器参数"() -> (w1172:T27)
                      n688 = Bundle By Name(cluster=w1172, "曲线截距"=w1169, "曲线斜率"=w1170, "二次多项式系数"=w1171) -> (w1173:T27)
                      n689 = global write "CODMn断电保存全局变量.vi" "CODMn仪器参数"(w1173) -> ()
                    }
                  }
                }
                frame Error {
                }
              }
            }
            n690 = One Button Dialog(message=w1148) -> ()  [unwired: 1 in, 1 out]
            n691 = control-ref of="量程下拉列表"() -> (w1145:refnum<vi>)
            n692 = local read "公式"() -> (w1144:cluster{"X^2":dbl, "X":dbl, "b":dbl})
            n693 = control-ref of="曲线模型"() -> (w1146:refnum<vi>)
            n694 = call "生成校准信息.vi"("table输入"="CODMn", "公式系数"=w1144, "量程下拉列表"=w1145, "曲线模型"=w1146) -> ()  [unwired: 8 in]
          }
        }
      }
      event "量程切换阈值读取": Value Change {
        n695 = event-data() -> ()  [unwired: 1 in, 6 out]
        n696 = property class="Enum (严格)"(reference=w1178) -> ("Value"=w1177:enum16{"CODMn"})  [unwired: 1 in, 2 out]
        n697 = call "量程读取.vi"("测量参数"=w1177) -> ("error out"=w1175:errorcluster)  [unwired: 9 in, 1 out]
        n698 = case shown="错误" w1175 {
          tunnel: ["读取成功" ("消息") "读取失败" ("消息")] -> w1176
          frame No Error {
          }
          frame Error {
          }
        }
        n699 = One Button Dialog(message=w1176) -> ()  [unwired: 1 in, 1 out]
      }
      event "量程切换阈值写入": Value Change {
        n700 = event-data() -> ()  [unwired: 1 in, 6 out]
        n701 = property class="Enum (严格)"(reference=w1184) -> ("Value"=w1183:enum16{"CODMn"})  [unwired: 1 in, 2 out]
        n702 = call "量程写入.vi"("测量参数"=w1183) -> ("error out"=w1181:errorcluster)  [unwired: 9 in]
        n703 = case shown="无错误" w1181 {
          tunnel: ["写入成功" ("消息") "写入失败" ("消息")] -> w1182
          frame No Error {
          }
          frame Error {
          }
        }
        n704 = One Button Dialog(message=w1182) -> ()  [unwired: 1 in, 1 out]
      }
    }
  }
  n705 = call "试剂余量后台任务.vi"() -> ()  [unwired: 12 in]
  n706 = while {
    tunnel: [w1194] -> _
    stop <- FALSE stop-if-true
    n707 = global read "VARCODMn全局变量.vi" "MB session in"() -> (w1195:refnum<class "MB_Master.lvclass">)
    n708 = control-ref of="试剂余量显示"() -> (w1198:refnum<vi>)
    n709 = Wait (ms)(milliseconds to wait=u32 10000 ("等待时间（毫秒）")) -> ()  [unwired: 1 out]
    n710 = call "试剂余量展示.vi"("波形图 2"=w1198) -> ("波形图"=→"试剂余量显示":sgl[][])  [unwired: 10 in]
    n711 = call "读取固件状态.vi"("MB session in"=w1195) -> ("error out"=w1194:errorcluster, "结果字符串"=w1190:string)  [unwired: 8 in, 1 out]
    n712 = Spreadsheet String To Array(delimiter (Tab)="\n" ("分隔符(Tab)"), format string="" ("格式字符串"), spreadsheet string=w1190, array type (2D Dbl)=string[] []) -> (array=w1189:string[])
    n713 = Index Array(array=w1189, index=1 ("索引")) -> (element=→"仪器版本号":string)
  }
